vi "Instrument Sequence.vi"(0 "Function":T5=enum."Initialize Dialog", 1 "Caller VI":enum16{"User", "Stress Measurement VI"}(ring), 2 "Which Program?":T1, 5 "Notifiers":T8, 7 "Message Queues":T21, 9 "Refnums":T6, 11 "error in (no error)":errorcluster, 12 "Configuration":variant) -> (8 "Instrument Steps":T2, 15 "error out":errorcluster)   [LabVIEW 2014]
uses:
  support/Message Queue/All Message Queues.ctl
  support/Message Queue/Message Cluster.ctl
  support/Notifiers/Notifiers.ctl
  support/Message Handler Loop Notifiers.ctl
  Hardware Control/Parameter Analyzer/Parameter Analyzer Notifiers.ctl
  Hardware Control/Switching Matrix/Switching Matrix Notifiers.ctl
  Hardware Control/Stress Control/StressControl Notifiers.ctl
  Hardware Control/Spectrometer/Spectrometer Notifiers.ctl
  Hardware Control/Switches and Mirrors/SwitchesMirrors Notifiers.ctl
  Hardware Control/Camera/Camera Notifiers.ctl
  Hardware Control/XYZ Stage/XYZ Notifications.ctl
  Hardware Control/Autofocus/Autofocus Notifiers.ctl
  Optoelectronic Measurement/Optoelectronic Notifiers.ctl
  Save Data/SaveData Notifiers.ctl
  Instrument Sequence Notifiers.ctl
  Instrument Sequence Refnums.ctl
  Action.ctl
  Instrument List.ctl
  Plot Data/Electrical Data Plot Refnums.ctl
  Instrument Sequence Function.ctl
  Instrument Steps.ctl
  Instrument Stequence - Which Program.ctl
  support/Status of All Instruments.ctl
  Hardware Control/Parameter Analyzer/Parameter Analyzer Data.ctl
  Hardware Control/Parameter Analyzer/Parameter Analyzer Config.ctl
  Hardware Control/Parameter Analyzer/Parameter Analyzer Integration Parameters.ctl
  Hardware Control/Parameter Analyzer/Parameter Analyzer SMU Sweeping.ctl
  Hardware Control/Parameter Analyzer/Parameter Analyzer Sweep Spacing.ctl
  Hardware Control/Parameter Analyzer/Parameter Analyzer SMU Range.ctl
  Hardware Control/Parameter Analyzer/Parameter Analyzer SMU Sampling.ctl
  Hardware Control/Parameter Analyzer/Parameter Analyzer Sampling Parameters.ctl
  Hardware Control/Parameter Analyzer/Parameter Analyzer Stop Sampling Conditions.ctl
  Hardware Control/Parameter Analyzer/Parameter Analyzer Refnums.ctl
  Hardware Control/Parameter Analyzer/Parameter Analyzer Initialization.ctl
  Hardware Control/Switching Matrix/Switching Matrix Data.ctl
  Hardware Control/Switching Matrix/Switching Matrix Config.ctl
  Hardware Control/Switching Matrix/Switching Matrix Refnums.ctl
  Hardware Control/Switching Matrix/Switching Matrix Initialization.ctl
  Hardware Control/Stress Control/StressControl Data.ctl
  Hardware Control/Stress Control/StressControl Config.ctl
  Hardware Control/Stress Control/StressControl Refnums.ctl
  Hardware Control/Stress Control/StressControl Initialization.ctl
  Hardware Control/Spectrometer/Spectrometer Data.ctl
  Hardware Control/Spectrometer/Spectrometer Config.ctl
  Hardware Control/Spectrometer/Laser Settings.ctl
  Hardware Control/Spectrometer/Laser.ctl
  Hardware Control/Spectrometer/Filter.ctl
  Hardware Control/Spectrometer/Grating Detector Settings.ctl
  Hardware Control/Spectrometer/Grating.ctl
  Hardware Control/Spectrometer/Detector.ctl
  Hardware Control/Spectrometer/Acquisition Settings.ctl
  Hardware Control/Spectrometer/Spectrometer Refnum.ctl
  Plot Data/Optical Spectrum Plot Refnum.ctl
  Hardware Control/Spectrometer/Spectrometer Initialization.ctl
  Hardware Control/Switches and Mirrors/SwitchesMirrors Data.ctl
  Hardware Control/Switches and Mirrors/SwitchesMirrors Config.ctl
  Hardware Control/Switches and Mirrors/SwitchesMirrors Status.ctl
  Hardware Control/Switches and Mirrors/SwitchesMirrors Refnum.ctl
  Hardware Control/Switches and Mirrors/SwitchesMirrors Initialize.ctl
  Hardware Control/Camera/Camera Data.ctl
  Hardware Control/Camera/Camera Config.ctl
  Hardware Control/Camera/Camera Settings.ctl
  Hardware Control/Camera/Camera Refnums.ctl
  Hardware Control/Camera/Camera Initialization.ctl
  Hardware Control/XYZ Stage/XYZ Data.ctl
  Hardware Control/XYZ Stage/XYZ Config.ctl
  Hardware Control/XYZ Stage/XYZ Connection Settings.ctl
  Hardware Control/XYZ Stage/XYZ Stage Control.ctl
  Hardware Control/XYZ Stage/XYZ Coordinate Control.ctl
  Hardware Control/XYZ Stage/XYZ Refnums.ctl
  Hardware Control/XYZ Stage/XYZ Initialization.ctl
  Hardware Control/Autofocus/AutoFocus Data.ctl
  Hardware Control/Autofocus/AutoFocus Config.ctl
  Hardware Control/Autofocus/ZScan.ctl
  <vilib>/Analysis/Matrix/Datatypes/RealMatrix.ctl
  Hardware Control/Autofocus/AutoFocus Refnums.ctl
  Hardware Control/Autofocus/Target Refnums.ctl
  Hardware Control/Autofocus/AutoFocus Initialize.ctl
  Hardware Control/Parameter Analyzer/Electrical Data.ctl
  Plot Data/WhichInstrument.ctl
  Hardware Control/Spectrometer/Spectral Data.ctl
  Optoelectronic Measurement/Optoelectronic Measurement.ctl
  <vilib>/Utility/sysdir.llb/System Directory Type.ctl
  support/Message Queue/Message Queue.lvlib
  <vilib>/Analysis/Matrix/NI_Matrix.lvlib
panel:
  out "Device Info":string
  out "Device Name":string
  # "LICENSED MATERIALS – PROPERTY OF IBM\nCopyright IBM Corp. 2016,\nALL RIGHTS RESERVED"
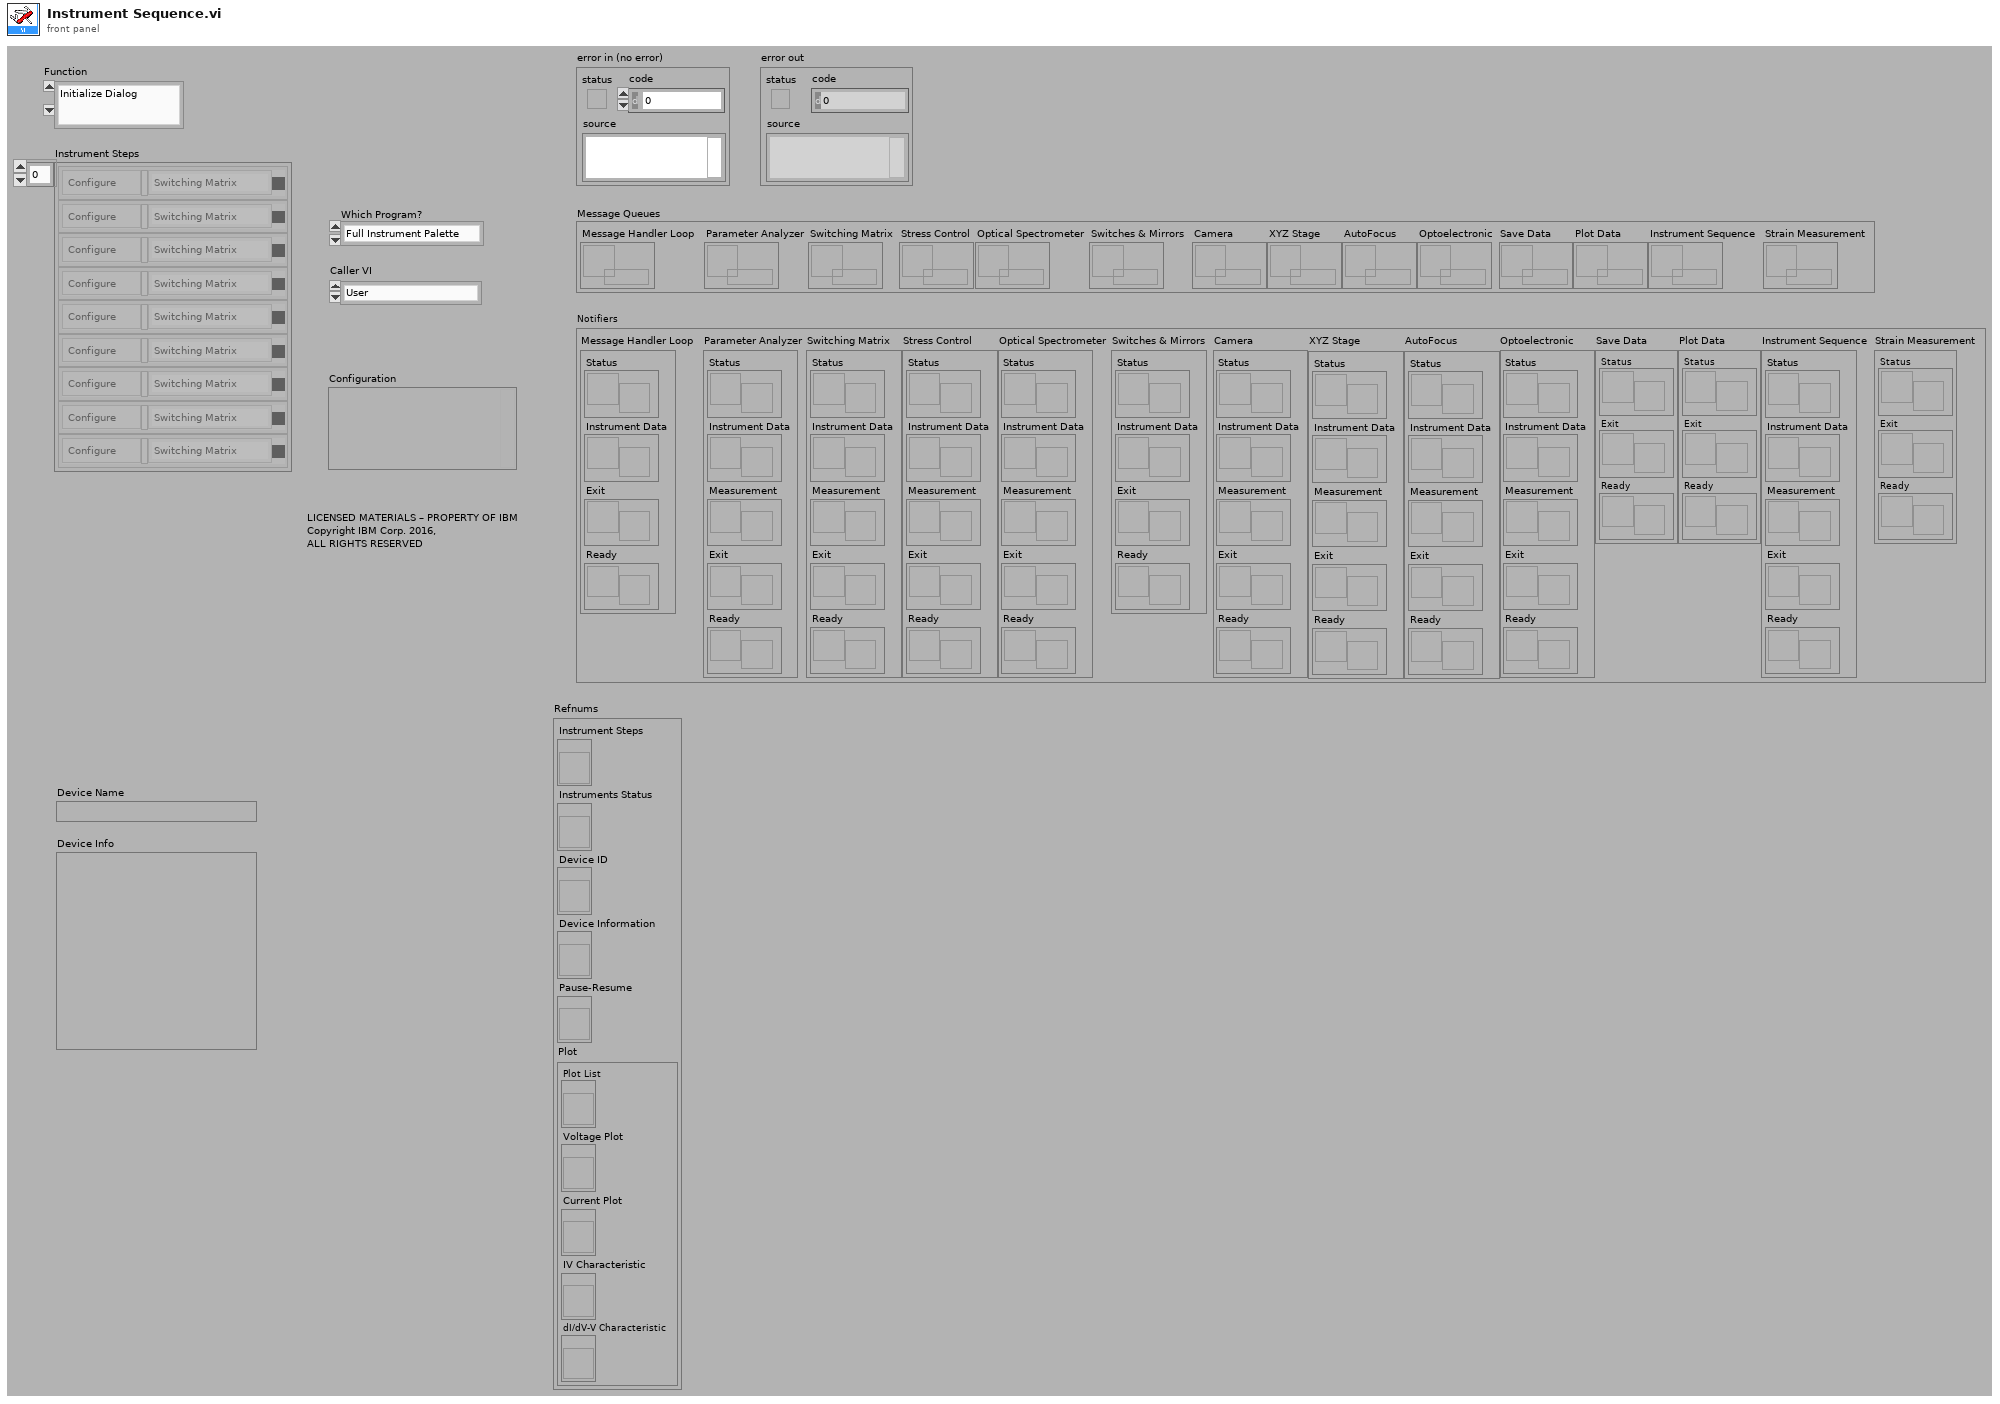
[diagram p1: front panel]
types:
  T1 = typedef "Instrument Stequence - Which Program.ctl" = enum16{"Full Instrument Palette", "Strain Electrical"}
  T2 = typedef "Instrument Steps.ctl" = cluster{"Action":T3, "Configuration":variant, "Instrument":T4, "Status":enum8{"False", "True", "Mixed"}}[]
  T3 = typedef "Action.ctl" = enum32{"Configure", "Measure"}
  T4 = typedef "Instrument List.ctl" = enum32{"Unknown Instrument", "Switching Matrix", "Parameter Analyzer", "Optical Spectrometer", "Optoelectronic", "Autofocus"}
  T5 = typedef "Instrument Sequence Function.ctl" = enum16{"Update Refnums", "Get Instruments Status", "Initialize Dialog", "Get Autofocus Status", "Add Step", "Remove Step", "Clear Sequence", "Load Sequence", "Save Sequence", "Measure Sequence", "Reset Sequence", "Start Sequence", "Start Sequence for Strain Measurement", "Stop Sequence", "Pause Sequence", "Update Sequence Status", "Choose What Next", "Update Workspace Data", "Save Measured Sequence", "Configure Parameter Analyzer", "Perform Electrical Measurement", "Configure Switching Matrix", "Configure Optical Spectrometer", "Focus", "Perform Optical Measurement", "Perform Optoelectronic Measurement", "Declare Completion"}
  T6 = typedef "Instrument Sequence Refnums.ctl" = cluster{"Instrument Steps":refnum<vi>, "Instruments Status":refnum<vi>, "Device ID":refnum<vi>, "Device Information":refnum<vi>, "Pause-Resume":refnum<vi>, "Plot":T7}
  T7 = typedef "Electrical Data Plot Refnums.ctl" = cluster{"Plot List":refnum<vi>, "Voltage Plot":refnum<vi>, "Current Plot":refnum<vi>, "IV Characteristic":refnum<vi>, "dI/dV-V Characteristic":refnum<vi>}
  T8 = typedef "Notifiers.ctl" = cluster{"Message Handler Loop":T9, "Parameter Analyzer":T10, "Switching Matrix":T11, "Stress Control":T12, "Optical Spectrometer":T13, "Switches & Mirrors":T14, "Camera":T15, "XYZ Stage":T16, "AutoFocus":T17, "Optoelectronic":T18, "Save Data":T19, "Plot Data":T19, "Instrument Sequence":T20, "Strain Measurement":cluster{"Status":refnum<notifier>, "Exit":refnum<notifier>, "Ready":refnum<notifier>}}
  T9 = typedef "Message Handler Loop Notifiers.ctl" = cluster{"Status":refnum<notifier>, "Instrument Data":refnum<notifier>, "Exit":refnum<notifier>, "Ready":refnum<notifier>}
  T10 = typedef "Parameter Analyzer Notifiers.ctl" = cluster{"Status":refnum<notifier>, "Instrument Data":refnum<notifier>, "Measurement":refnum<notifier>, "Exit":refnum<notifier>, "Ready":refnum<notifier>}
  T11 = typedef "Switching Matrix Notifiers.ctl" = cluster{"Status":refnum<notifier>, "Instrument Data":refnum<notifier>, "Measurement":refnum<notifier>, "Exit":refnum<notifier>, "Ready":refnum<notifier>}
  T12 = typedef "StressControl Notifiers.ctl" = cluster{"Status":refnum<notifier>, "Instrument Data":refnum<notifier>, "Measurement":refnum<notifier>, "Exit":refnum<notifier>, "Ready":refnum<notifier>}
  T13 = typedef "Spectrometer Notifiers.ctl" = cluster{"Status":refnum<notifier>, "Instrument Data":refnum<notifier>, "Measurement":refnum<notifier>, "Exit":refnum<notifier>, "Ready":refnum<notifier>}
  T14 = typedef "SwitchesMirrors Notifiers.ctl" = cluster{"Status":refnum<notifier>, "Instrument Data":refnum<notifier>, "Exit":refnum<notifier>, "Ready":refnum<notifier>}
  T15 = typedef "Camera Notifiers.ctl" = cluster{"Status":refnum<notifier>, "Instrument Data":refnum<notifier>, "Measurement":refnum<notifier>, "Exit":refnum<notifier>, "Ready":refnum<notifier>}
  T16 = typedef "XYZ Notifications.ctl" = cluster{"Status":refnum<notifier>, "Instrument Data":refnum<notifier>, "Measurement":refnum<notifier>, "Exit":refnum<notifier>, "Ready":refnum<notifier>}
  T17 = typedef "Autofocus Notifiers.ctl" = cluster{"Status":refnum<notifier>, "Instrument Data":refnum<notifier>, "Measurement":refnum<notifier>, "Exit":refnum<notifier>, "Ready":refnum<notifier>}
  T18 = typedef "Optoelectronic Notifiers.ctl" = cluster{"Status":refnum<notifier>, "Instrument Data":refnum<notifier>, "Measurement":refnum<notifier>, "Exit":refnum<notifier>, "Ready":refnum<notifier>}
  T19 = typedef "SaveData Notifiers.ctl" = cluster{"Status":refnum<notifier>, "Exit":refnum<notifier>, "Ready":refnum<notifier>}
  T20 = typedef "Instrument Sequence Notifiers.ctl" = cluster{"Status":refnum<notifier>, "Instrument Data":refnum<notifier>, "Measurement":refnum<notifier>, "Exit":refnum<notifier>, "Ready":refnum<notifier>}
  T21 = typedef "Message Queue.lvlib/All Message Queues.ctl" = cluster{"Message Handler Loop":refnum<queue>, "Parameter Analyzer":refnum<queue>, "Switching Matrix":refnum<queue>, "Stress Control":refnum<queue>, "Optical Spectrometer":refnum<queue>, "Switches & Mirrors":refnum<queue>, "Camera":refnum<queue>, "XYZ Stage":refnum<queue>, "AutoFocus":refnum<queue>, "Optoelectronic":refnum<queue>, "Save Data":refnum<queue>, "Plot Data":refnum<queue>, "Instrument Sequence":refnum<queue>, "Strain Measurement":refnum<queue>}
  T22 = typedef "WhichInstrument.ctl" = enum16{"No Plot", "Spectrometer", "Parameter Analyzer", "Optoelectronic"}
  T23 = typedef "Electrical Data.ctl" = cluster{"Sequence":dbl[], "V1":dbl[], "V2":dbl[], "V3":dbl[], "V4":dbl[], "I1":dbl[], "I2":dbl[], "I3":dbl[], "I4":dbl[]}
  T24 = typedef "Spectral Data.ctl" = cluster{"Intensity":dbl[], "Wavelength":dbl[], "Energy":dbl[], "Raman Shift":dbl[], "Detector Temperature":dbl}
  T25 = typedef "Optoelectronic Measurement.ctl" = cluster{"Optical Spectrum":T24, "Electrical Measurement":T23}
  T26 = typedef "Parameter Analyzer Data.ctl" = cluster{"Configuration":T27, "Refnums":T35, "Initialization":T36}
  T27 = typedef "Parameter Analyzer Config.ctl" = cluster{"Parameter Analyzer VISA Session":refnum<visa-resource-name>, "Sweeping Time Parameters":T28, "Acquisition Mode":enum32{"Sweeping Mode", "Sampling Mode"}, "Status Polling Time (ms)":u32, "Comment":string, "SMU 1 - Sweeping":T29, "SMU 2 - Sweeping":T29, "SMU 3 - Sweeping":T29, "SMU 4 - Sweeping":T29, "Sweep Spacing":T30, "Range":T31, "SMU1 - Sampling":T32, "SMU2 - Sampling":T32, "SMU3 - Sampling":T32, "SMU4 - Sampling":T32, "Sampling Time Parameters":T33, "Stop Condition":T34}
  T28 = typedef "Parameter Analyzer Integration Parameters.ctl" = cluster{"Integration Time":u32, "Short Integration Time (s)":dbl, "Long Integration Time (s)":dbl, "Wait Time Parameter":dbl}
  T29 = typedef "Parameter Analyzer SMU Sweeping.ctl" = cluster{"Start / Offset":dbl, "Stop / Ratio":dbl, "Step \n(linear only)":dbl, "Compliance":dbl, "Power \nCompliance":dbl, "Mode":u32, "Function":i32, "Sweep Mode":bool}
  T30 = typedef "Parameter Analyzer Sweep Spacing.ctl" = u16
  T31 = typedef "Parameter Analyzer SMU Range.ctl" = u16
  T32 = typedef "Parameter Analyzer SMU Sampling.ctl" = cluster{"Source":dbl, "Compliance":dbl, "Mode":u32, "Function":bool}
  T33 = typedef "Parameter Analyzer Sampling Parameters.ctl" = cluster{"Initial Interval (s)":dbl, "Number of Samples":i32, "Total Sampling Time (s)":dbl, "Hold Time (s)":dbl, "Sampling Mode":i32, "Sampling Time":i32}
  T34 = typedef "Parameter Analyzer Stop Sampling Conditions.ctl" = cluster{"Enable Delay (s)":dbl, "Name":string, "Threshold":dbl, "num. of events":i32, "Event":i32, "Stop Condition Enable":bool}
  T35 = typedef "Parameter Analyzer Refnums.ctl" = cluster{"Status":refnum<vi>, "Electrical Measurement":refnum<vi>, "Plots":T7, "HP Integration Time":refnum<vi>, "VISA":refnum<vi>, "Sweeping Time Parameters":refnum<vi>, "Acquisition Mode":refnum<vi>, "SMU 1 - Sweeping":refnum<vi>, "SMU 2 - Sweeping":refnum<vi>, "SMU 3 - Sweeping":refnum<vi>, "SMU 4 - Sweeping":refnum<vi>, "Sweep Spacing":refnum<vi>, "Range":refnum<vi>, "SMU1 - Sampling":refnum<vi>, "SMU2 - Sampling":refnum<vi>, "SMU3 - Sampling":refnum<vi>, "SMU4 - Sampling":refnum<vi>, "Sampling Time Parameters":refnum<vi>, "Stop Condition":refnum<vi>, "Instrument Status":refnum<vi>}
  T36 = typedef "Parameter Analyzer Initialization.ctl" = cluster{"Update Visa Session":bool, "Configure Integration Time":bool, "Configure Acquisition Mode":bool, "Update Refnums":bool}
  T37 = typedef "Switching Matrix Data.ctl" = cluster{"Configuration":T38, "Refnums":T39, "Initialization":T40}
  T38 = typedef "Switching Matrix Config.ctl" = cluster{"Switching Matrix VISA Session":refnum<visa-resource-name>, "Connections":cluster{"Connections":bool[], "Connection Type":enum16{"Disconnected", "Make - Break", "Break - Make"}}[]}
  T39 = typedef "Switching Matrix Refnums.ctl" = cluster{"Connections":refnum<vi>, "Instrument Status":refnum<vi>}
  T40 = typedef "Switching Matrix Initialization.ctl" = cluster{"Update Visa Session":bool, "Update Refnums":bool}
  T41 = typedef "Spectrometer Data.ctl" = cluster{"Configuration":T42, "Refnums":T50, "Initialization":T52}
  T42 = typedef "Spectrometer Config.ctl" = cluster{"Laser Settings":T43, "Spectrometer Settings":T46, "Acquisition Settings":T49, "Path":path}
  T43 = typedef "Laser Settings.ctl" = cluster{"Laser Wavelength":T44, "Neutral Density Filter":T45}
  T44 = typedef "Laser.ctl" = enum16{"633 nm", "784 nm", "532 nm", "365 nm"}
  T45 = typedef "Filter.ctl" = enum16{"100%", "50%", "25%", "10%", "1%", "0.1%", "0.01%"}
  T46 = typedef "Grating Detector Settings.ctl" = cluster{"Confocal Hole Size (µm)":dbl, "Grating":T47, "Detector":T48}
  T47 = typedef "Grating.ctl" = u16
  T48 = typedef "Detector.ctl" = enum16{"InGaAs Array", "Silicon CCD"}
  T49 = typedef "Acquisition Settings.ctl" = cluster{"Acquisition Mode":enum16{"Single Window", "Multi-Window"}, "Spectal Position (nm)":dbl, "From (nm)":dbl, "To (nm)":dbl, "Integration Time (s)":dbl, "Number of Accumulations":i32, "AutoScanning":bool, "Spike Removal":bool}
  T50 = typedef "Spectrometer Refnum.ctl" = cluster{"Instrument Status":refnum<vi>, "Optical Spectrum Plot":T51, "Laser":refnum<vi>, "Filter":refnum<vi>, "Laser ON?":refnum<vi>, "Hole":refnum<vi>, "Grating":refnum<vi>, "Detector":refnum<vi>, "Acquisition Mode":refnum<vi>, "Spectal Position":refnum<vi>, "From":refnum<vi>, "To":refnum<vi>, "Integration Time":refnum<vi>, "Accumulations":refnum<vi>, "AutoScanning":refnum<vi>, "Spike Removal":refnum<vi>, "Acquisition Mode Panel":refnum<vi>}
  T51 = typedef "Optical Spectrum Plot Refnum.ctl" = cluster{"Plot List":refnum<vi>, "Optical Spectrum vs Energy":refnum<vi>, "Optical Spectrum vs Wavelength":refnum<vi>, "Optical Spectrum vs Raman Shift":refnum<vi>, "Detector Temperature":refnum<vi>}
  T52 = typedef "Spectrometer Initialization.ctl" = cluster{"Connect":bool, "Update Refnums":bool, "Get Configuration":bool}
  T53 = typedef "AutoFocus Data.ctl" = cluster{"Configuration":T54, "Refnums":T57, "Initialize":T59}
  T54 = typedef "AutoFocus Config.ctl" = cluster{"Matching Criteria":cluster{"Minimum Score":sgl, "Color Score Weight":sgl, "Minimum Contrast":i32, "Match Mode":u32, "Match Feature Mode":u32, "Subpixel Accuracy":bool, "Color Sensitivity":u32, "Search Strategy":u32}, "Z Scan Parameters":T55, "Displacement":dbl, "Transformation Matrix":T56}
  T55 = typedef "ZScan.ctl" = cluster{"Z Range":ext, "Resolution":dbl, "Initial Direction":enum16{"Up", "Down"}, "Focus Threshold":dbl, "Ascent Constant":dbl}
  T56 = typedef "NI_Matrix.lvlib/RealMatrix.ctl" = dbl[][]
  T57 = typedef "AutoFocus Refnums.ctl" = cluster{"Instrument Status":refnum<vi>, "Matching Criteria":refnum<vi>, "Z Scan Parameters":refnum<vi>, "Distance":refnum<vi>, "Transformation Matrix":refnum<vi>, "Match and Edge":T58, "Matching Curves":refnum<vi>, "Tracking":refnum<vi>, "Focus":refnum<vi>, "Find Focus":refnum<vi>, "Set Target":refnum<vi>, "Link Stage & Camera":refnum<vi>, "Align":refnum<vi>}
  T58 = typedef "Target Refnums.ctl" = cluster{"Image":refnum<vi>, "Target":refnum<vi>, "Edge":refnum<vi>, "Target Data":refnum<vi>}
  T59 = typedef "AutoFocus Initialize.ctl" = cluster{"Update Refnums":bool, "Allocate Image Memory":bool, "Set Match Criteria":bool, "Link Stage & Camera":bool, "Set Target":bool, "Find Target":bool}
  T60 = typedef "Status of All Instruments.ctl" = cluster{"Parameter Analyzer":T26, "Swithing Matrix":T37, "Stress Control":T61, "Optical Spectrometer":T41, "Switches & Mirrors":T65, "Camera":T70, "XYZ Stage":T75, "AutoFocus":T53}
  T61 = typedef "StressControl Data.ctl" = cluster{"Configuration":T62, "Refnums":T63, "Initialization":T64}
  T62 = typedef "StressControl Config.ctl" = cluster{"Stress Control VISA Session":refnum<visa-resource-name>, "Axis":i32, "Motion":u16, "Destination (°)":dbl, "Speed (°/s)":dbl, "Position (°)":dbl}
  T63 = typedef "StressControl Refnums.ctl" = cluster{"Instrument Status":refnum<vi>, "Position":refnum<vi>, "Mecahnism Motion":refnum<vi>, "Destination":refnum<vi>, "Apply Stress":refnum<vi>, "Stop":refnum<vi>, "Stress Control VISA":refnum<vi>}
  T64 = typedef "StressControl Initialization.ctl" = cluster{"Update Visa Session":bool, "Update Configuration":bool, "Update Refnums":bool, "Get Position":bool}
  T65 = typedef "SwitchesMirrors Data.ctl" = cluster{"Configuration":T66, "Refnums":T68, "Initialize":T69}
  T66 = typedef "SwitchesMirrors Config.ctl" = cluster{"Relay VISA Session":refnum<visa-resource-name>, "Switches":T67, "Delays (ms)":cluster{"Laser":u32, "Video":u32}}
  T67 = typedef "SwitchesMirrors Status.ctl" = cluster{"Laser":bool, "Video":bool}
  T68 = typedef "SwitchesMirrors Refnum.ctl" = cluster{"Instrument Status":refnum<vi>, "Laser":refnum<vi>, "Video":refnum<vi>, "Relay VISA":refnum<vi>}
  T69 = typedef "SwitchesMirrors Initialize.ctl" = cluster{"Update Refnums":bool, "Connect":bool, "Set Configuration":bool}
  T70 = typedef "Camera Data.ctl" = cluster{"Configuration":T71, "Refnums":T73, "Initialization":T74}
  T71 = typedef "Camera Config.ctl" = cluster{"Settings":T72}
  T72 = typedef "Camera Settings.ctl" = cluster{"Pixel clock":i32, "Frame rate":dbl, "Exposure time":dbl, "Master Gain":i32, "Red Gain":i32, "Green Gain":i32, "Blue Gain":i32, "Auto Gain":bool, "White-balance":bool, "Color Correction":bool}
  T73 = typedef "Camera Refnums.ctl" = cluster{"Pixel Clock":refnum<vi>, "Frame Rate":refnum<vi>, "Exposure Time":refnum<vi>, "Master Gain":refnum<vi>, "Red Gain":refnum<vi>, "Green Gain":refnum<vi>, "Blue Gain":refnum<vi>, "Auto Gain":refnum<vi>, "Auto White-balance":refnum<vi>, "Color Correction":refnum<vi>, "Image":refnum<vi>, "Video Button":refnum<vi>, "Instrument Status":refnum<vi>}
  T74 = typedef "Camera Initialization.ctl" = cluster{"Connect":bool, "Update Refnums":bool, "Acquiring?":bool}
  T75 = typedef "XYZ Data.ctl" = cluster{"Configuration":T76, "Refnums":T80, "Initialization":T81}
  T76 = typedef "XYZ Config.ctl" = cluster{"Connection Settings":T77, "Manual Control":T78, "Coordinate Control":T79}
  T77 = typedef "XYZ Connection Settings.ctl" = cluster{"Tango VISA":refnum<visa-resource-name>, "Baudrate":i32, "Show Protocol?":bool}
  T78 = typedef "XYZ Stage Control.ctl" = cluster{"North":bool, "South":bool, "West":bool, "East":bool, "Up":bool, "Down":bool, "Stop":bool, "XY Step":dbl, "Z step":dbl}
  T79 = typedef "XYZ Coordinate Control.ctl" = cluster{"Motion Mode":enum16{"Absolute", "Relative"}, "Destination [mm]":dbl[]}
  T80 = typedef "XYZ Refnums.ctl" = cluster{"Instrument Status":refnum<vi>, "Position":refnum<vi>, "Manual Control":refnum<vi>, "Up":refnum<vi>, "Down":refnum<vi>, "North":refnum<vi>, "South":refnum<vi>, "East":refnum<vi>, "West":refnum<vi>, "Stop":refnum<vi>, "Limits":refnum<vi>}
  T81 = typedef "XYZ Initialization.ctl" = cluster{"Update Visa Session":bool, "Set To Default":bool, "Get Status":bool, "Update Refnums":bool}
  T82 = typedef "System Directory Type.ctl" = i32
  T83 = cluster{"Action":T3, "Configuration":variant, "Instrument":T4, "Status":enum8{"False", "True", "Mixed"}}
  T84 = typedef "SaveData Workspace Info.ctl" = cluster{"Device Name":string, "Device Info":string, "Path":path}
  T85 = typedef "Measurement.ctl" = cluster{"Which Instrument?":T22, "Electrical Measurement":T23, "Measurement Mode":enum16{"Sweeping Mode", "Sampling Mode"}, "Optical Spectrum":T24}
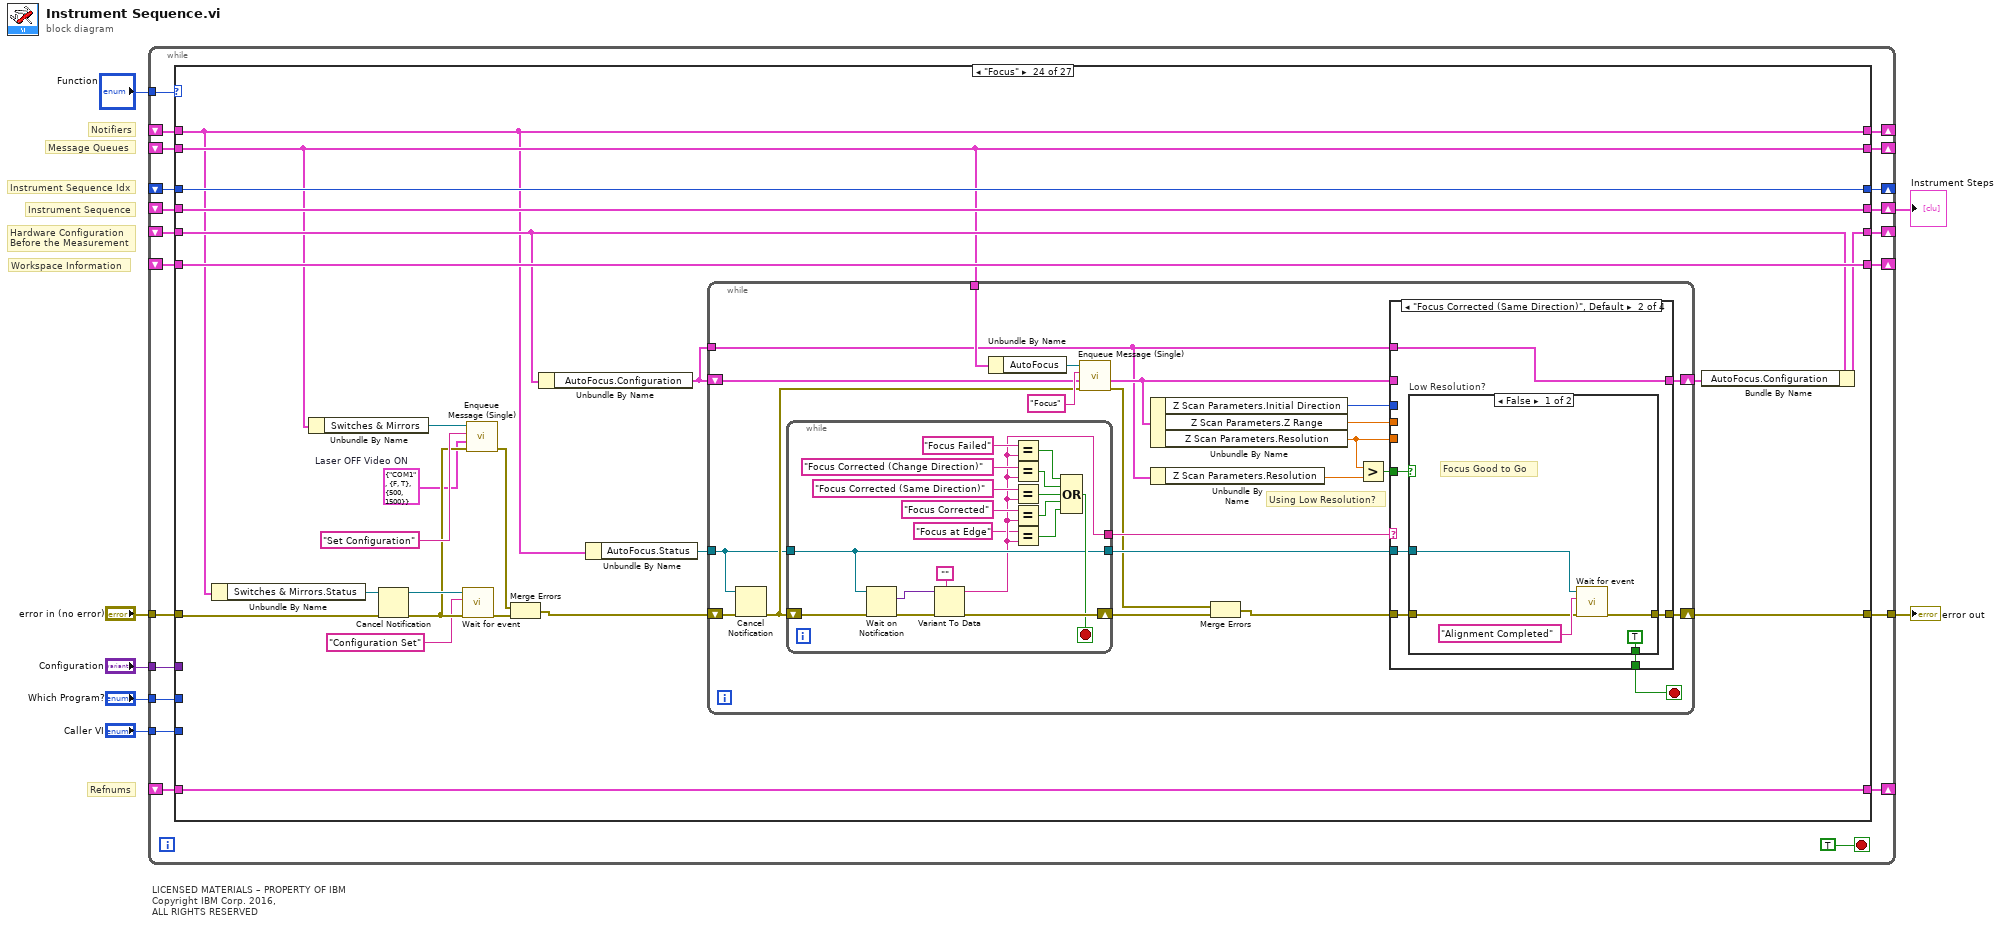
[diagram p0: block diagram]
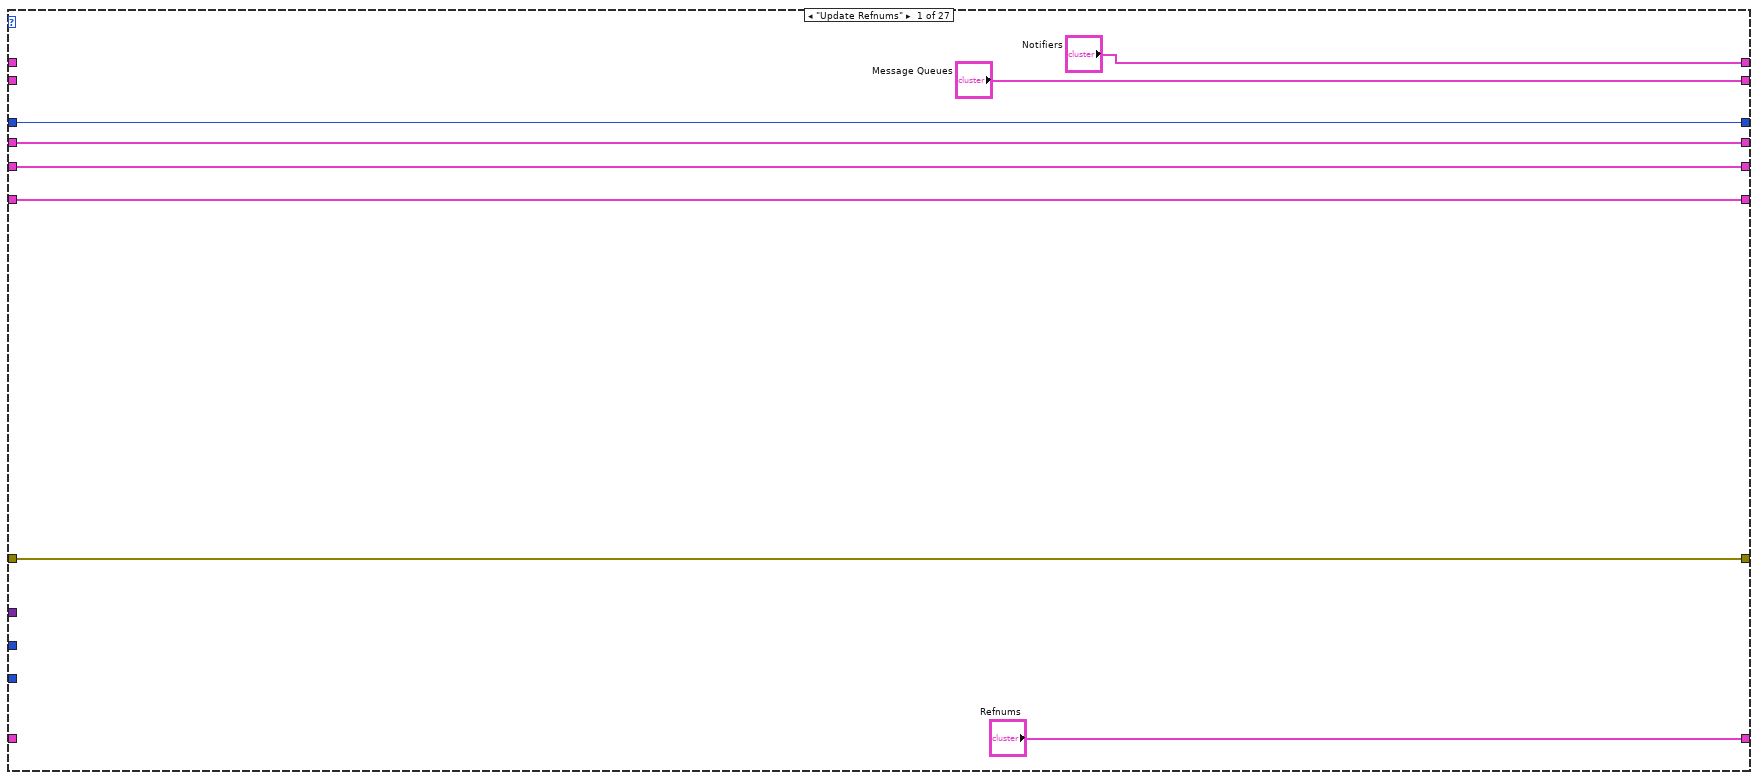
[diagram p2: hidden frame]
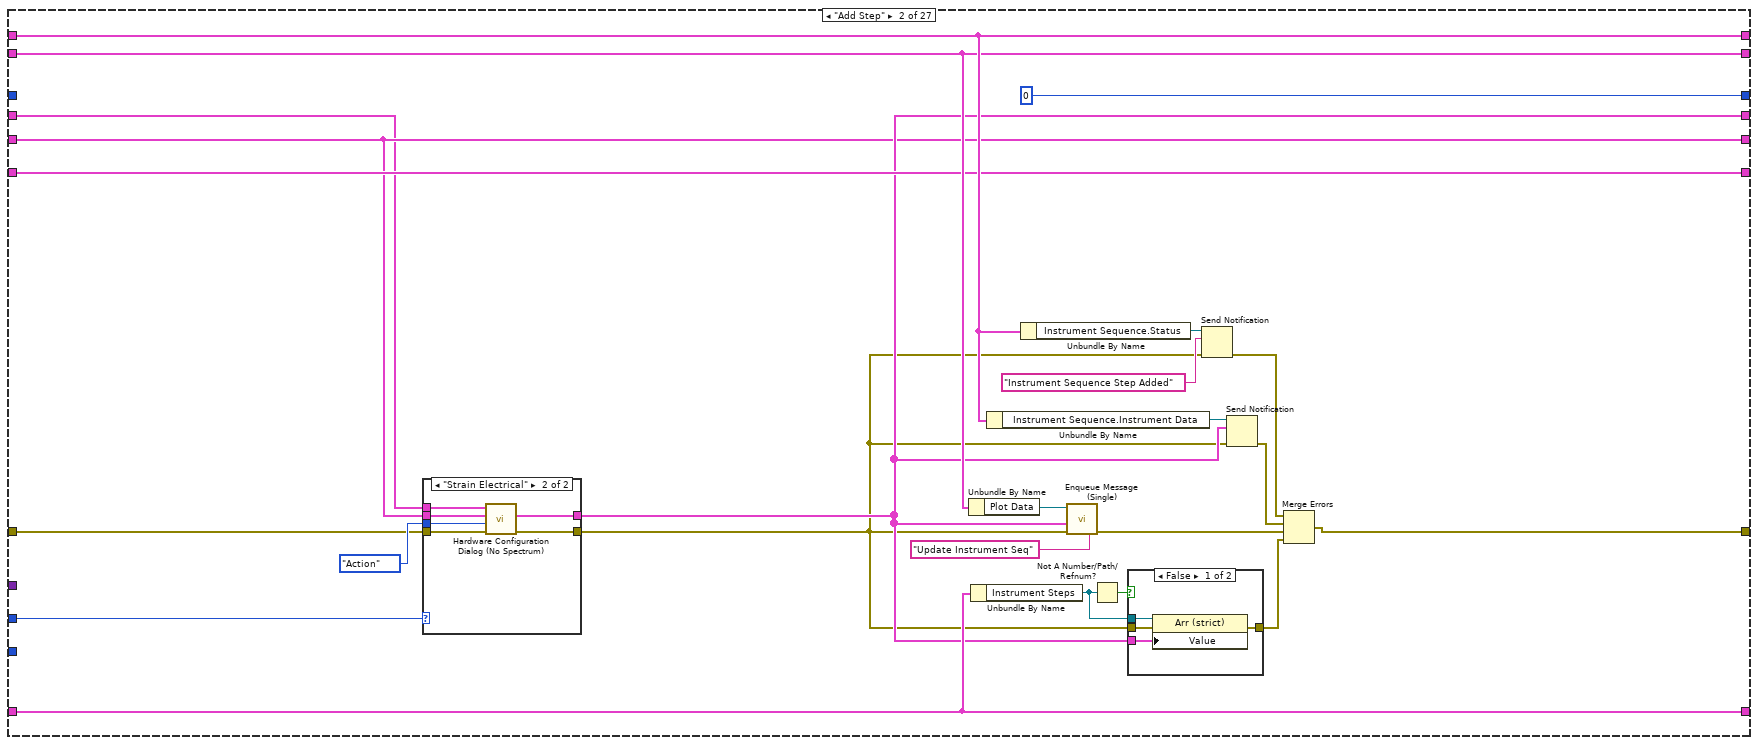
[diagram p3: hidden frame]
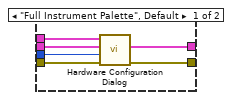
[diagram p4: hidden frame]
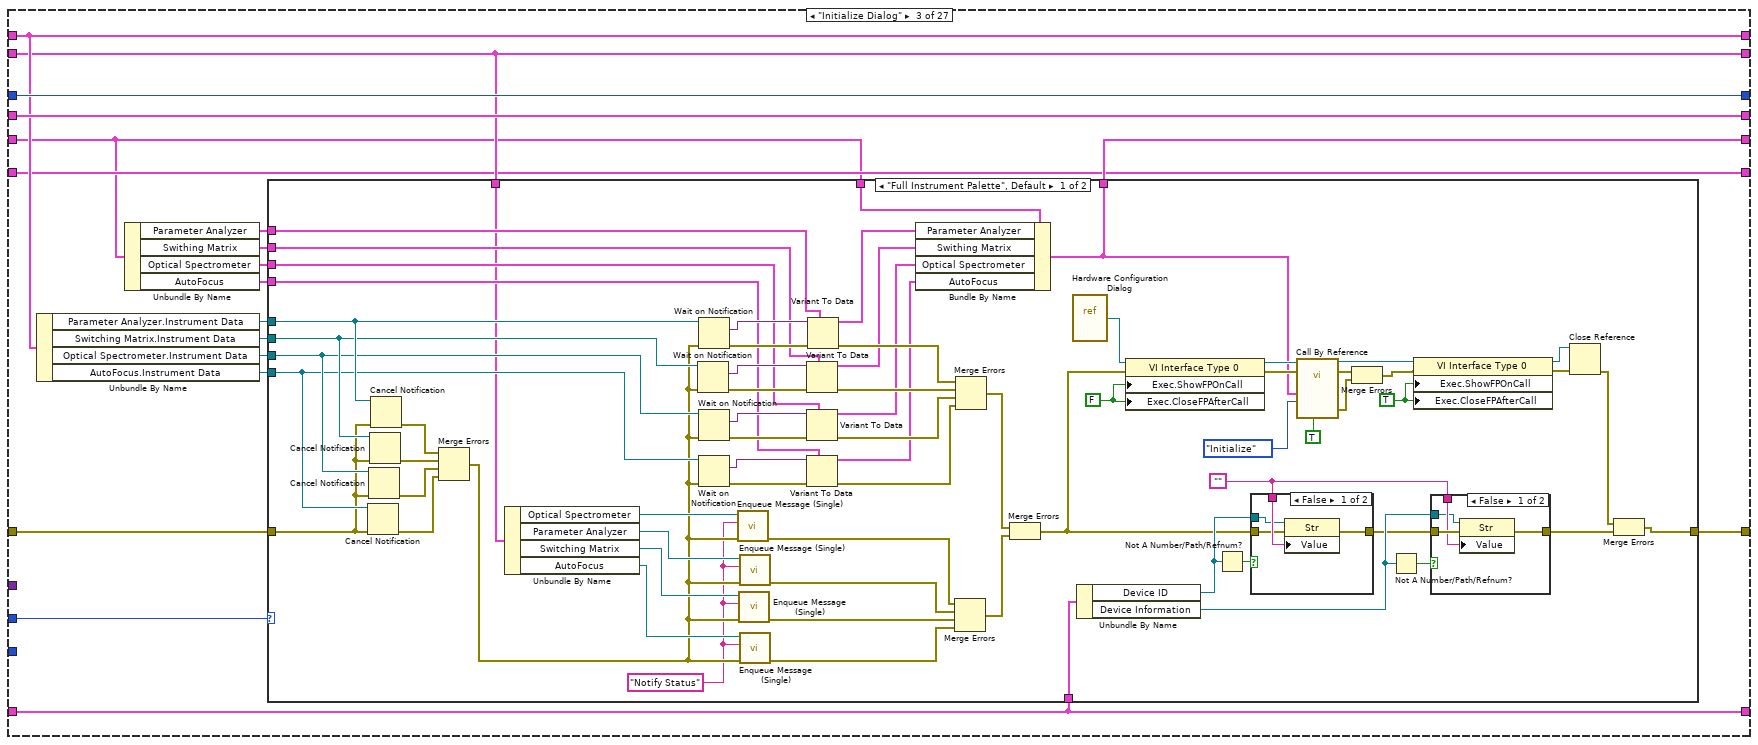
[diagram p6: hidden frame]
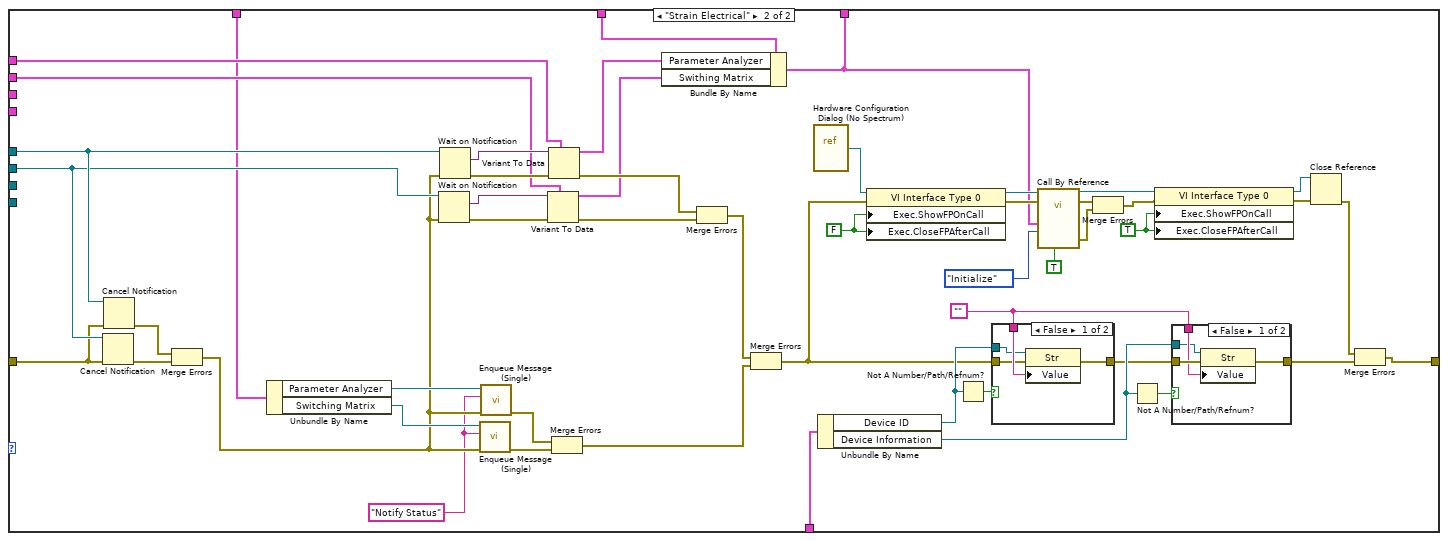
[diagram p9: hidden frame]
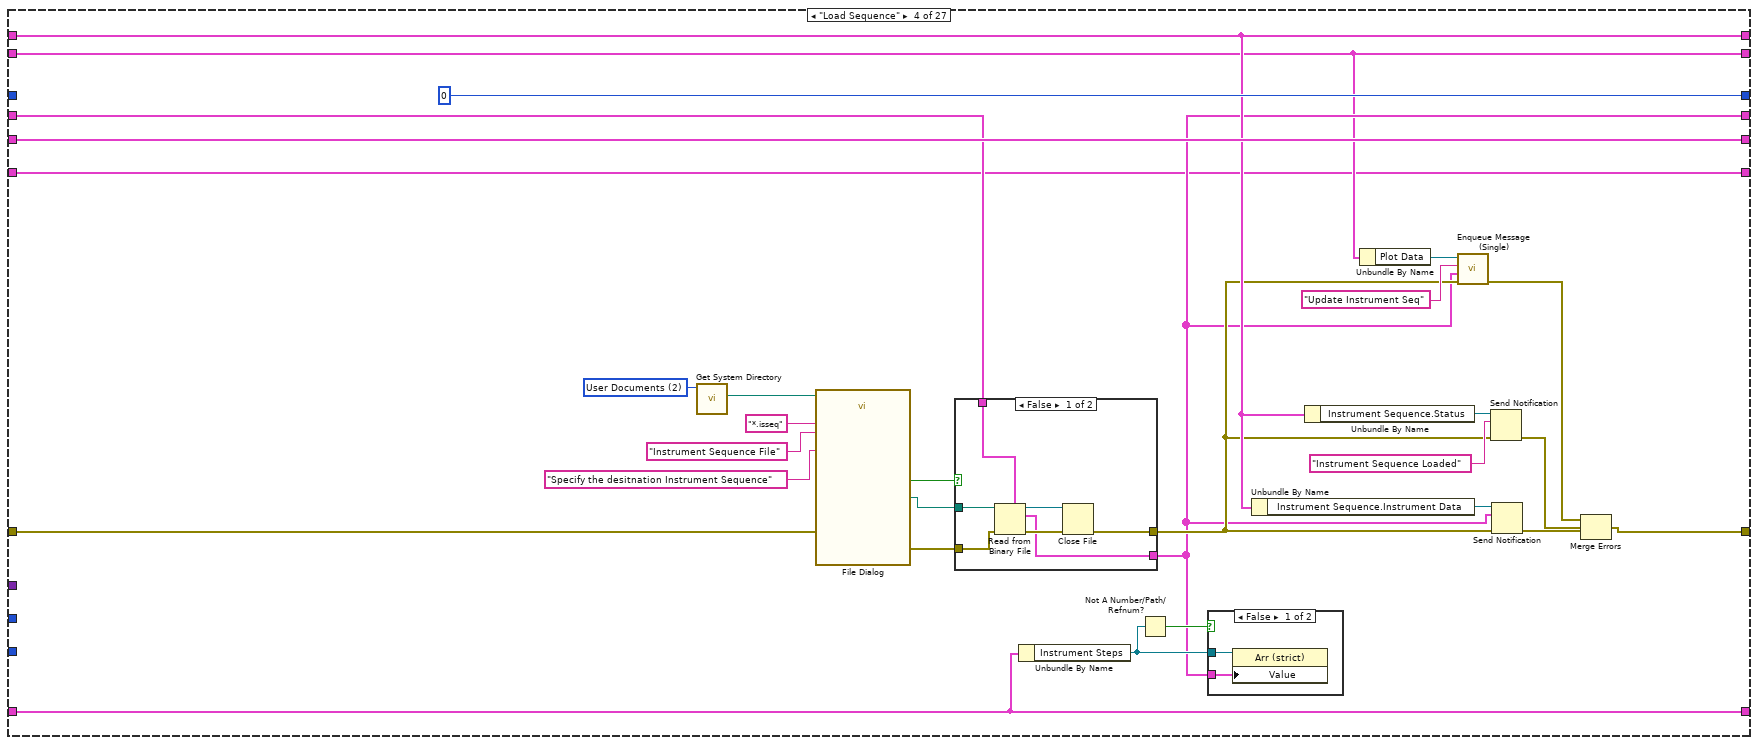
[diagram p12: hidden frame]
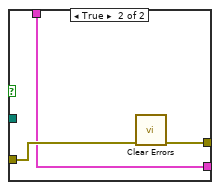
[diagram p13: hidden frame]
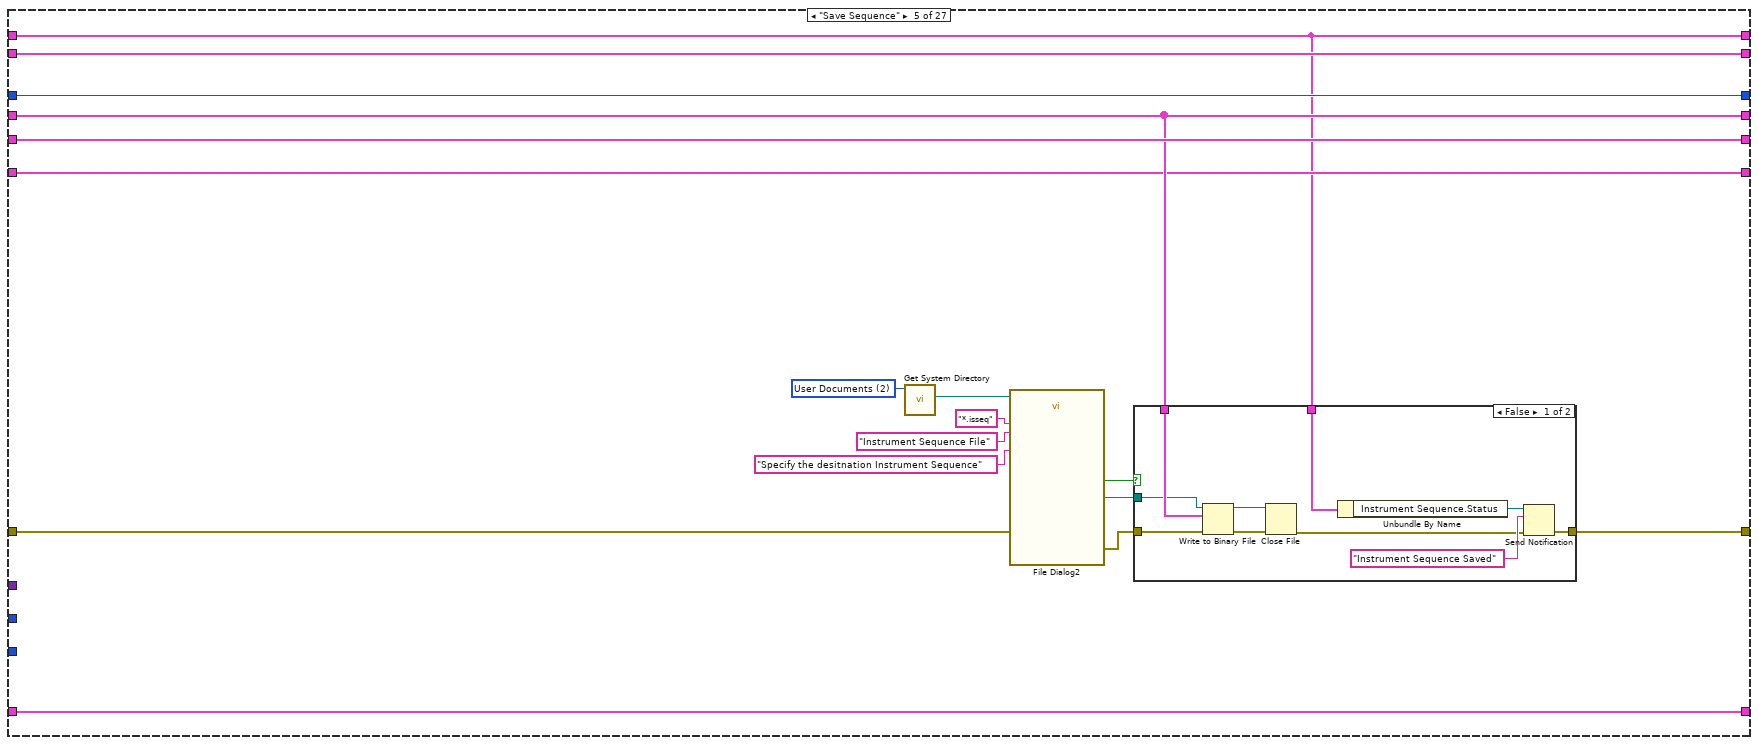
[diagram p15: hidden frame]
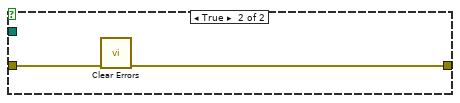
[diagram p16: hidden frame]
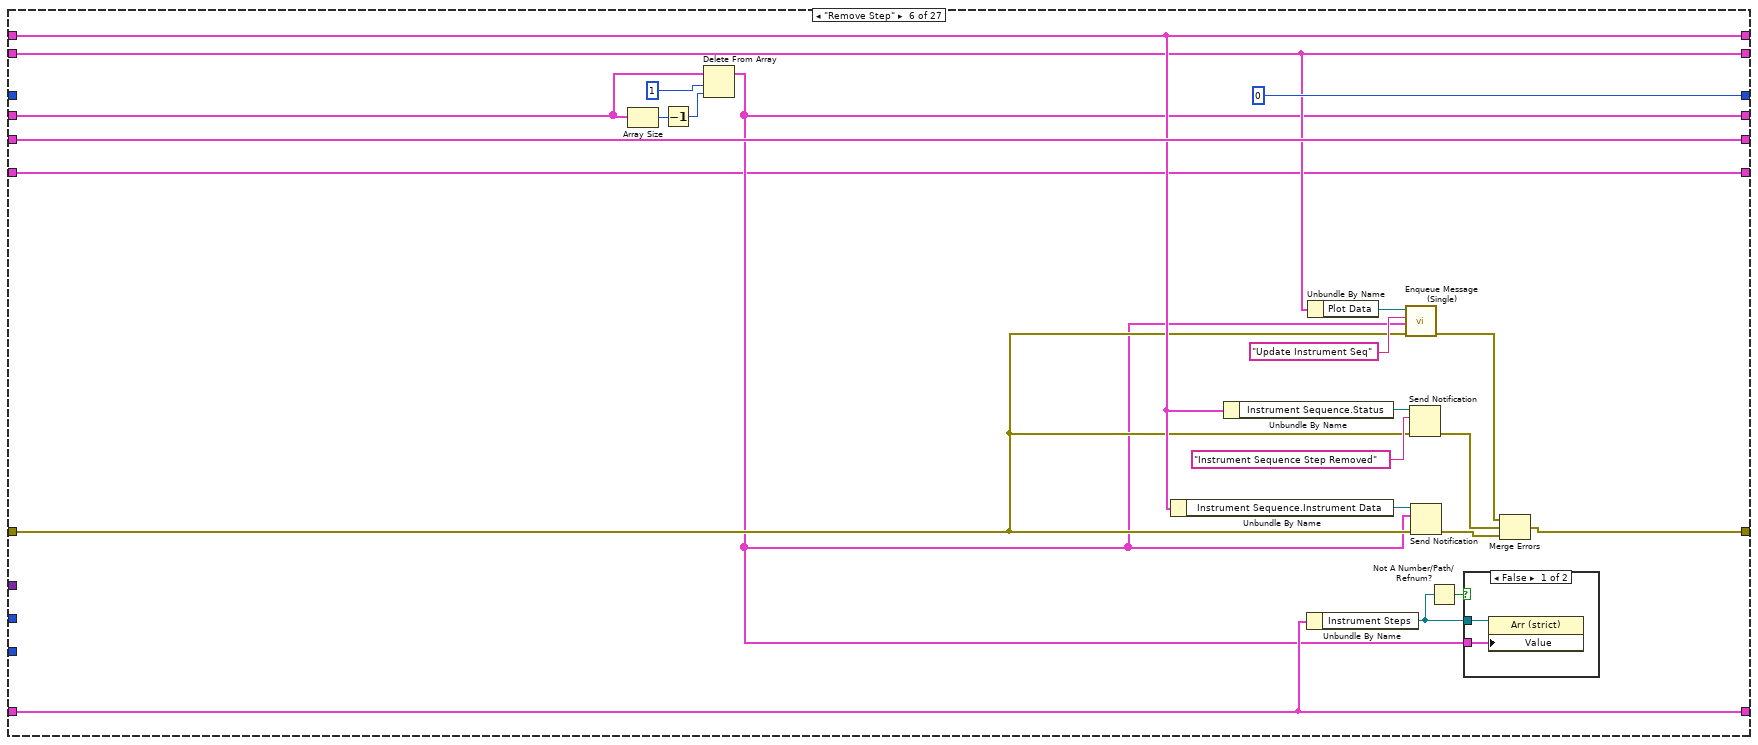
[diagram p17: hidden frame]
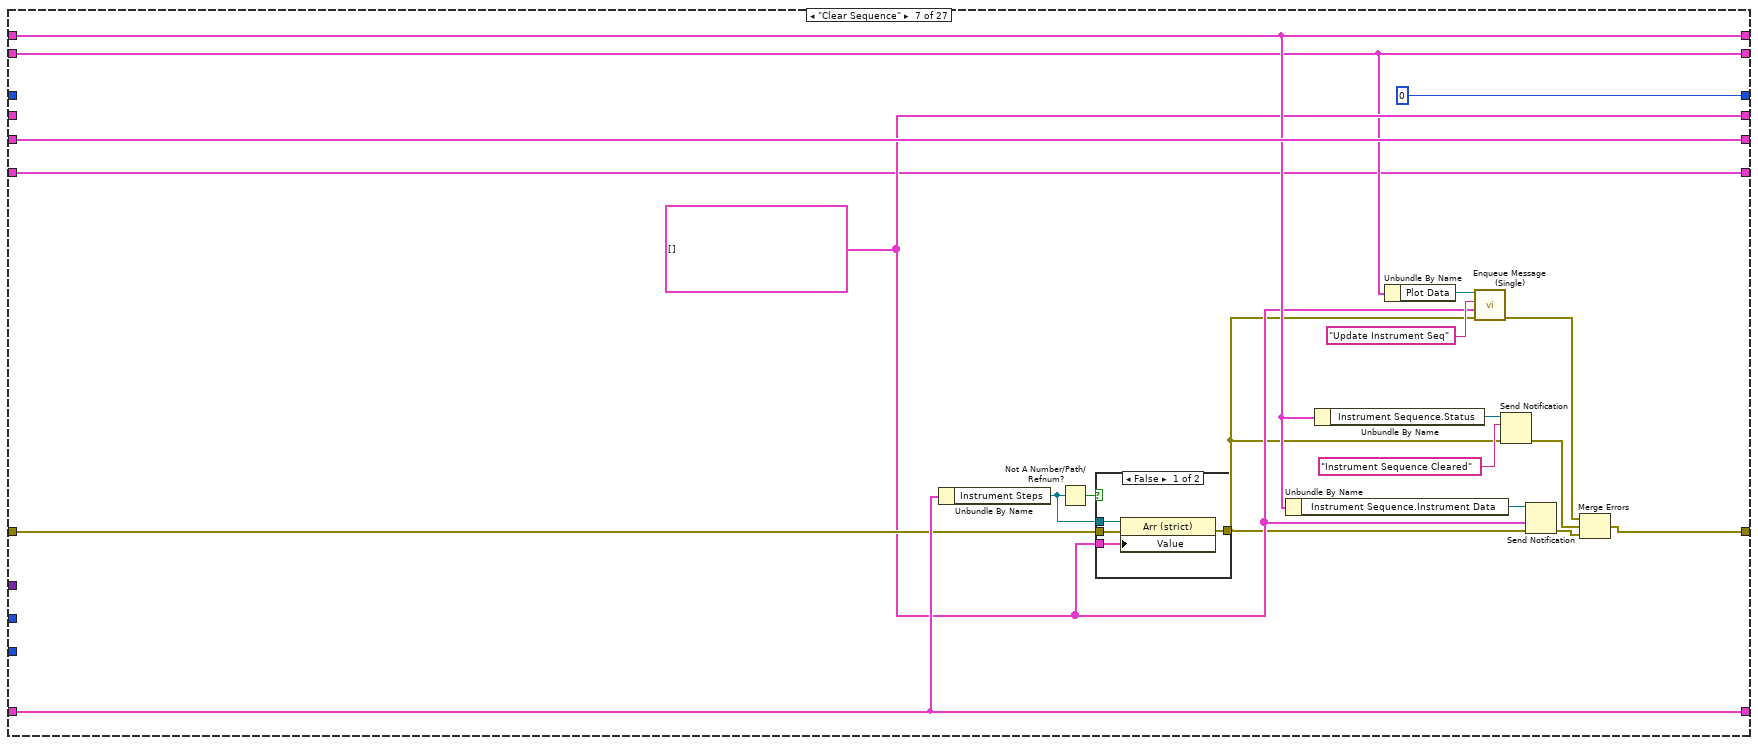
[diagram p19: hidden frame]
diagram:
  # "LICENSED MATERIALS – PROPERTY OF IBM\nCopyright IBM Corp. 2016,\nALL RIGHTS RESERVED"
  # "Workspace Information"
  # "Instrument Sequence Idx"
  # "Instrument Sequence"
  # "Refnums"
  # "Hardware Configuration\nBefore the Measurement"
  # "Message Queues"
  # "Notifiers"
  n1 = while {
    tunnel: "error in (no error)" -> [w28]
    tunnel: [w27] -> w6
    tunnel: "Function" -> [w26]
    shift-right: [w21] -> _
    shift-left: _ -> [w22]
    shift-right: [w20] -> _
    shift-left: _ -> [w25]
    shift-right: [w19] -> _
    shift-left: _ -> [w24]
    shift-right: [w17] -> _
    shift-left: _ -> [w18]
    shift-right: [w16] -> w4
    shift-left: _ -> [w15]
    shift-right: [w13] -> _
    shift-left: _ -> [w14]
    tunnel: "Configuration" -> [w12]
    tunnel: "Caller VI" -> [w11]
    shift-right: [w9] -> _
    shift-left: _ -> [w10]
    tunnel: "Which Program?" -> [w8]
    stop <- TRUE stop-if-true
    n2 = case shown="\"Focus\"" w26 {
      tunnel: w28 -> [w36 w38 w82 w256 w284 w307 w339 w380 w388 w408 w481 w519 w550 w597 w631 w648 w749 w763 w816 w897 w957 w993 w1024 w1057 w1170 w1179 w1189]
      tunnel: [w36 w44 w93 w246 w278 w314 w340 w372 w387 w411 w487 w513 w551 w593 w627 w661 w738 w776 w835 w914 w967 w1005 w1041 w1049 w1165 w1177 w1190] -> w27
      tunnel: w25 -> [_ w51 w83 w249 w279 w315 w341 w359 w400 w421 w486 w512 w540 w598 w633 w659 w754 w790 w832 w911 w969 w987 w1018 w1050 w1174 w1184 w1187]
      tunnel: w24 -> [_ w48 w81 w238 w291 w309 w334 w358 w391 w406 w496 w526 w544 w590 w642 w658 w753 w765 w834 w913 w965 w1003 w1039 w1051 w1168 w1183 w1197]
      tunnel: ["Refnums" w57 w94 w260 w290 w323 w345 w386 w401 w422 w483 w522 w546 w594 w638 w660 w755 w796 w865 w940 w968 w1007 w1043 w1068 w1169 w1178 w1193] -> w21
      tunnel: w22 -> [_ w57 w94 w260 w290 w323 w345 w386 w401 w422 w483 w522 w546 w594 w638 w660 w755 w796 w865 w940 w968 w1007 w1043 w1068 w1169 w1178 w1193]
      tunnel: ["Notifiers" w51 w83 w249 w279 w315 w341 w359 w400 w421 w486 w512 w540 w598 w633 w659 w754 w790 w832 w911 w969 w987 w1018 w1050 w1174 w1184 w1187] -> w20
      tunnel: ["Message Queues" w48 w81 w238 w291 w309 w334 w358 w391 w406 w496 w526 w544 w590 w642 w658 w753 w765 w834 w913 w965 w1003 w1039 w1051 w1168 w1183 w1197] -> w19
      tunnel: w18 -> [w32 w40 w79 w263 w292 w327 w349 w385 w399 w420 w494 w525 w541 w587 w641 _ w741 w778 w805 w889 w974 w1011 w1046 w1054 w1171 w1180 w1194]
      tunnel: [w32 w40 w84 w263 w292 w327 w349 w385 w399 w420 w494 w525 w541 w587 w641 w657 w752 w778 w805 w889 w961 w1000 w1036 w1053 w1171 w1180 w1194] -> w17
      tunnel: [w30 w43 w96 w242 w288 w306 w336 w384 w398 w419 w482 w511 w545 w589 w639 w652 w751 w795 w863 w938 w977 w1012 w1047 w1070 w1172 w1181 w1195] -> w16
      tunnel: w15 -> [w30 w39 w96 w253 w288 w319 _ w384 w398 w419 w495 w510 w545 w589 w639 w652 w751 w795 w863 w938 w977 w1012 w1047 w1070 w1172 w1181 w1195]
      tunnel: w14 -> [w31 _ w95 _ w289 _ _ w383 w397 w418 _ w509 w548 _ w640 w651 w750 w794 w862 w937 w978 w1013 w1048 w1071 w1173 w1182 w1196]
      tunnel: [w31 0 w95 0 w289 0 0 w383 w397 w418 0 w509 w547 0 w640 w651 w750 w794 w862 w937 w978 w1013 w1048 w1071 w1173 w1182 w1196] -> w13
      tunnel: w12 -> [_ _ _ _ _ _ _ _ _ _ _ _ _ _ _ _ _ _ _ _ w966 w1006 w1042 _ _ _ _]
      tunnel: w11 -> [_ _ _ _ _ _ _ _ _ w402 _ _ w543 _ _ _ _ _ _ _ _ _ _ _ _ _ w1188]
      tunnel: w10 -> [w29 w47 w80 w237 w280 w305 w330 w379 w395 w403 w479 w505 w542 _ w635 w644 w742 w775 w833 w912 w959 w999 w1029 w1067 w1166 w1175 w1185]
      tunnel: [w29 w47 w80 w237 w280 w305 w330 w379 w395 w403 w479 w505 w542 w588 w635 w644 w742 w775 w833 w912 w959 w999 w1029 w1067 w1166 w1175 w1185] -> w9
      tunnel: w8 -> [_ w37 w78 _ _ _ _ _ _ _ _ _ _ _ _ w643 _ _ _ _ _ _ _ _ _ _ _]
      frame "Update Refnums" {
      }
      frame "Add Step" {
        n3 = case shown="\"Strain Electrical\"" w37 {
          tunnel: [w66 w72] -> w43
          tunnel: [w65 w71] -> w42
          tunnel: enum16{"Initialize", "Action"}."Action" ("Function") -> [w64 w70]
          tunnel: w40 -> [w63 w69]
          tunnel: w39 -> [w62 w68]
          tunnel: w38 -> [w61 w67]
          frame "Full Instrument Palette", Default {
            n4 = call "Hardware Configuration Dialog.vi"("error in (no error)"=w61, "Function"=w64, "Hardware Status"=w63, "Instrument Steps In"=w62) -> ("error out"=w65:errorcluster, "Instrument Steps Out"=w66:T2)  [unwired: 6 in]
          }
          frame "Strain Electrical" {
            n5 = call "Hardware Configuration Dialog (No Spectrum).vi"("error in (no error)"=w67, "Function"=w70, "Hardware Status"=w69, "Instrument Steps In"=w68) -> ("error out"=w71:errorcluster, "Instrument Steps Out"=w72:T2)  [unwired: 6 in]
          }
        }
        n6 = Unbundle By Name(w48) -> ("Plot Data"=w50:refnum<queue>)
        n7 = Unbundle By Name(w57) -> ("Instrument Steps"=w58:refnum<vi>)
        n8 = Unbundle By Name(w51) -> ("Instrument Sequence.Instrument Data"=w54:refnum<notifier>)
        n9 = Unbundle By Name(w51) -> ("Instrument Sequence.Status"=w55:refnum<notifier>)
        n10 = call "Enqueue Message (Single).vi"("error in (no error)"=w42, "Message Data"=w43, "Message"="Update Instrument Seq", "Message Queue"=w50) -> ("error out"=w45:errorcluster)  [unwired: 7 out]
        n11 = Not A Number/Path/Refnum?(number/path/refnum=w58) -> (NaN/Path/Refnum?=w59:bool)
        n12 = case shown="False" w59 {
          tunnel: w58 -> [w76 _]
          tunnel: w43 -> [w75 _]
          tunnel: w42 -> [w74 w77]
          tunnel: [w73 w77] -> w46
          frame False {
            n13 = property class="Arr (strict)"(reference=w76, error in=w74, "Value"=w75) -> (error out=w73:errorcluster)  [unwired: 1 out]
          }
          frame True {
          }
        }
        n14 = Send Notification(notification="Instrument Sequence Step Added", notifier=w55, error in (no error)=w42) -> (error out=w52:errorcluster)  [unwired: 1 out]
        n15 = Send Notification(notification=w43, notifier=w54, error in (no error)=w42) -> (error out=w53:errorcluster)  [unwired: 1 out]
        n16 = Merge Errors(w52, w53, w45, w46) -> (w44:errorcluster)
      }
      frame "Initialize Dialog" {
        n17 = Unbundle By Name(w83) -> ("Parameter Analyzer.Instrument Data"=w90:refnum<notifier>, "Switching Matrix.Instrument Data"=w89:refnum<notifier>, "Optical Spectrometer.Instrument Data"=w88:refnum<notifier>, "AutoFocus.Instrument Data"=w86:refnum<notifier>)
        n18 = Unbundle By Name(w79) -> ("Parameter Analyzer"=w92:T26, "Swithing Matrix"=w91:T37, "Optical Spectrometer"=w87:T41, "AutoFocus"=w85:T53)
        n19 = case shown="\"Full Instrument Palette\", Default" w78 {
          tunnel: w94 -> [w158 w218]
          tunnel: [w143 w203] -> w93
          tunnel: w92 -> [w134 w195]
          tunnel: w91 -> [w133 w194]
          tunnel: w90 -> [w131 w192]
          tunnel: w89 -> [w130 w191]
          tunnel: w88 -> [w119 _]
          tunnel: w87 -> [w118 _]
          tunnel: w86 -> [w114 _]
          tunnel: w85 -> [w111 _]
          tunnel: [w97 w175] -> w84
          tunnel: w82 -> [w101 w179]
          tunnel: w81 -> [w100 w178]
          tunnel: w79 -> [w98 w176]
          frame "Full Instrument Palette", Default {
            w104 = "Notify Status" ("Message")
            w149 = TRUE ("Execution:Show Front Panel On Call")
            w150 = FALSE ("Execution:Show Front Panel On Call")
            w157 = "" ("Device Name")
            n20 = Cancel Notification(0:w114, 3:w101) -> (11:w115:errorcluster)  [unwired: 2 out]
            n21 = Cancel Notification(0:w119, 3:w101) -> (11:w123:errorcluster)  [unwired: 2 out]
            n22 = Cancel Notification(0:w130, 3:w101) -> (11:w129:errorcluster)  [unwired: 2 out]
            n23 = Cancel Notification(0:w131, 3:w101) -> (11:w128:errorcluster)  [unwired: 2 out]
            n24 = Merge Errors(w128, w129, w123, w115) -> (w105:errorcluster)
            n25 = Unbundle By Name(w100) -> ("Optical Spectrometer"=w109:refnum<queue>, "Parameter Analyzer"=w108:refnum<queue>, "Switching Matrix"=w107:refnum<queue>, "AutoFocus"=w106:refnum<queue>)
            n26 = Wait on Notification(notifier=w130, error in (no error)=w105) -> (notification=w135:variant, error out=w136:errorcluster)  [unwired: 4 out]
            n27 = Wait on Notification(notifier=w131, error in (no error)=w105) -> (notification=w141:variant, error out=w140:errorcluster)  [unwired: 4 out]
            n28 = Wait on Notification(notifier=w119, error in (no error)=w105) -> (notification=w120:variant, error out=w122:errorcluster)  [unwired: 4 out]
            n29 = Wait on Notification(notifier=w114, error in (no error)=w105) -> (notification=w113:variant, error out=w112:errorcluster)  [unwired: 4 out]
            n30 = call "Enqueue Message (Single).vi"("error in (no error)"=w105, "Message"=w104, "Message Queue"=w109) -> ("error out"=w103:errorcluster)  [unwired: 1 in, 7 out]
            n31 = call "Enqueue Message (Single).vi"("error in (no error)"=w105, "Message"=w104, "Message Queue"=w107) -> ("error out"=w138:errorcluster)  [unwired: 1 in, 7 out]
            n32 = call "Enqueue Message (Single).vi"("error in (no error)"=w105, "Message"=w104, "Message Queue"=w108) -> ("error out"=w139:errorcluster)  [unwired: 1 in, 7 out]
            n33 = call "Enqueue Message (Single).vi"("error in (no error)"=w105, "Message"=w104, "Message Queue"=w106) -> ("error out"=w137:errorcluster)  [unwired: 1 in, 7 out]
            n34 = Variant To Data(error in=w136, type=w133, Variant=w135) -> (data=w116:T37, error out=w126:errorcluster)
            n35 = Variant To Data(error in=w122, type=w118, Variant=w120) -> (data=w117:T41, error out=w121:errorcluster)
            n36 = Variant To Data(error in=w112, type=w111, Variant=w113) -> (data=w102:T53, error out=w110:errorcluster)
            n37 = Variant To Data(error in=w140, type=w134, Variant=w141) -> (data=w132:T26, error out=w127:errorcluster)
            n38 = Bundle By Name(cluster=w98, "Parameter Analyzer"=w132, "Swithing Matrix"=w116, "Optical Spectrometer"=w117, "AutoFocus"=w102) -> (w97:T60)
            n39 = Merge Errors(w103, w139, w138, w137) -> (w124:errorcluster)
            n40 = Merge Errors(w127, w126, w121, w110) -> (w125:errorcluster)
            n41 = Merge Errors(w125, w124) -> (w99:errorcluster)
            n42 = vi-ref "Hardware Configuration Dialog.vi"() -> (w148:refnum<vi>)
            n43 = Unbundle By Name(w158) -> ("Device ID"=w162:refnum<vi>, "Device Information"=w164:refnum<vi>)
            n44 = property class="VI Interface Type 0"(reference=w148, error in=w99, "Exec.ShowFPOnCall"=w150, "Exec.CloseFPAfterCall"=w150) -> (reference out=w144:refnum<vi>, error out=w145:errorcluster)
            n45 = Not A Number/Path/Refnum?(number/path/refnum=w162) -> (NaN/Path/Refnum?=w161:bool)
            n46 = case shown="False" w161 {
              tunnel: [w173 w174] -> w160
              tunnel: w157 -> [w172 _]
              tunnel: w162 -> [w171 _]
              tunnel: w99 -> [w170 w174]
              frame False {
                n47 = property class="Str"(reference=w171, error in=w170, "Value"=w172) -> (error out=w173:errorcluster)  [unwired: 1 out]
              }
              frame True {
              }
            }
            n48 = call-by-ref "?"(reference=w144, error in=w145, "Update UI Values?"=TRUE, "Function"=enum16{"Initialize", "Action"}."Initialize", "Hardware Status"=w97) -> (reference out=w147:refnum<vi>, error out=w153:errorcluster, 0:"error out"=w156:errorcluster)  [unwired: 7 in, 1 out]
            n49 = Merge Errors(w153, w156) -> (w146:errorcluster)
            n50 = Not A Number/Path/Refnum?(number/path/refnum=w164) -> (NaN/Path/Refnum?=w163:bool)
            n51 = property class="VI Interface Type 0"(reference=w147, error in=w146, "Exec.ShowFPOnCall"=w149, "Exec.CloseFPAfterCall"=w149) -> (reference out=w151:refnum<vi>, error out=w152:errorcluster)
            n52 = case shown="False" w163 {
              tunnel: w160 -> [w168 w169]
              tunnel: [w167 w169] -> w159
              tunnel: w157 -> [w166 _]
              tunnel: w164 -> [w165 _]
              frame False {
                n53 = property class="Str"(reference=w165, error in=w168, "Value"=w166) -> (error out=w167:errorcluster)  [unwired: 1 out]
              }
              frame True {
              }
            }
            n54 = Close Reference(reference=w151, error in (no error)=w152) -> (error out=w142:errorcluster)
            n55 = Merge Errors(w142, w159) -> (w143:errorcluster)
          }
          frame "Strain Electrical" {
            w180 = "Notify Status" ("Message")
            w209 = TRUE ("Execution:Show Front Panel On Call")
            w210 = FALSE ("Execution:Show Front Panel On Call")
            w217 = "" ("Device Name")
            n56 = Cancel Notification(0:w191, 3:w179) -> (11:w190:errorcluster)  [unwired: 2 out]
            n57 = Cancel Notification(0:w192, 3:w179) -> (11:w189:errorcluster)  [unwired: 2 out]
            n58 = Merge Errors(w189, w190) -> (w181:errorcluster)
            n59 = Unbundle By Name(w178) -> ("Parameter Analyzer"=w183:refnum<queue>, "Switching Matrix"=w182:refnum<queue>)
            n60 = Wait on Notification(notifier=w191, error in (no error)=w181) -> (notification=w196:variant, error out=w197:errorcluster)  [unwired: 4 out]
            n61 = Wait on Notification(notifier=w192, error in (no error)=w181) -> (notification=w201:variant, error out=w200:errorcluster)  [unwired: 4 out]
            n62 = call "Enqueue Message (Single).vi"("error in (no error)"=w181, "Message"=w180, "Message Queue"=w182) -> ("error out"=w198:errorcluster)  [unwired: 1 in, 7 out]
            n63 = call "Enqueue Message (Single).vi"("error in (no error)"=w181, "Message"=w180, "Message Queue"=w183) -> ("error out"=w199:errorcluster)  [unwired: 1 in, 7 out]
            n64 = Variant To Data(error in=w197, type=w194, Variant=w196) -> (data=w184:T37, error out=w187:errorcluster)
            n65 = Variant To Data(error in=w200, type=w195, Variant=w201) -> (data=w193:T26, error out=w188:errorcluster)
            n66 = Merge Errors(w199, w198) -> (w185:errorcluster)
            n67 = Bundle By Name(cluster=w176, "Parameter Analyzer"=w193, "Swithing Matrix"=w184) -> (w175:T60)
            n68 = Merge Errors(w188, w187) -> (w186:errorcluster)
            n69 = Merge Errors(w186, w185) -> (w177:errorcluster)
            n70 = vi-ref "Hardware Configuration Dialog (No Spectrum).vi"() -> (w208:refnum<vi>)
            n71 = Unbundle By Name(w218) -> ("Device ID"=w222:refnum<vi>, "Device Information"=w224:refnum<vi>)
            n72 = property class="VI Interface Type 0"(reference=w208, error in=w177, "Exec.ShowFPOnCall"=w210, "Exec.CloseFPAfterCall"=w210) -> (reference out=w204:refnum<vi>, error out=w205:errorcluster)
            n73 = Not A Number/Path/Refnum?(number/path/refnum=w222) -> (NaN/Path/Refnum?=w221:bool)
            n74 = case shown="False" w221 {
              tunnel: [w233 w234] -> w220
              tunnel: w217 -> [w232 _]
              tunnel: w222 -> [w231 _]
              tunnel: w177 -> [w230 w234]
              frame False {
                n75 = property class="Str"(reference=w231, error in=w230, "Value"=w232) -> (error out=w233:errorcluster)  [unwired: 1 out]
              }
              frame True {
              }
            }
            n76 = call-by-ref "?"(reference=w204, error in=w205, "Update UI Values?"=TRUE, "Function"=enum16{"Initialize", "Action"}."Initialize", "Hardware Status"=w175) -> (reference out=w207:refnum<vi>, error out=w213:errorcluster, 0:"error out"=w216:errorcluster)  [unwired: 7 in, 1 out]
            n77 = Merge Errors(w213, w216) -> (w206:errorcluster)
            n78 = Not A Number/Path/Refnum?(number/path/refnum=w224) -> (NaN/Path/Refnum?=w223:bool)
            n79 = property class="VI Interface Type 0"(reference=w207, error in=w206, "Exec.ShowFPOnCall"=w209, "Exec.CloseFPAfterCall"=w209) -> (reference out=w211:refnum<vi>, error out=w212:errorcluster)
            n80 = case shown="False" w223 {
              tunnel: w220 -> [w228 w229]
              tunnel: [w227 w229] -> w219
              tunnel: w217 -> [w226 _]
              tunnel: w224 -> [w225 _]
              frame False {
                n81 = property class="Str"(reference=w225, error in=w228, "Value"=w226) -> (error out=w227:errorcluster)  [unwired: 1 out]
              }
              frame True {
              }
            }
            n82 = Close Reference(reference=w211, error in (no error)=w212) -> (error out=w202:errorcluster)
            n83 = Merge Errors(w202, w219) -> (w203:errorcluster)
          }
        }
      }
      frame "Load Sequence" {
        w236 = T82 2 items=["User Home"=0, "User Desktop"=1, "User Documents"=2, "User Application Data"=3, "User Preferences"=4, "User Temporary"=5, "Public Documents"=6, "Public Application Data"=7, "Public Preferences"=8, "Public Cache"=13, "System Core Libraries"=9, "System Installed Libraries"=10, "Application Files"=11, "Boot Volume Root"=12] ("system directory type")
        n84 = call <vilib>:"Get System Directory.vi"("system directory type"=w236) -> ("system directory"=w235:path)  [unwired: 10 in]
        n85 = call "File Dialog"("start path"=w235, "prompt"="Specify the desitnation Instrument Sequence", "error in"=w256, "pattern (all files)"="*.isseq", "pattern label"="Instrument Sequence File") -> ("selected path"=w252:path, "cancelled"=w255:bool, "error out"=w254:errorcluster)  [unwired: 2 in, 6 out]
        n86 = case shown="False" w255 {
          tunnel: w254 -> [w270 w273]
          tunnel: [w265 w271] -> w243
          tunnel: w253 -> [w268 w272]
          tunnel: [w267 w272] -> w242
          tunnel: w252 -> [w266 _]
          frame False {
            n87 = Read from Binary File(5:w268, 8:w270, 11:w266) -> (0:w269:errorcluster, 2:w267:T2, 3:w264:refnum<file>)  [unwired: 1 in, 3 out]
            n88 = Close File(refnum=w264, error in=w269) -> (error out=w265:errorcluster)  [unwired: 1 out]
          }
          frame True {
            n89 = call <vilib>:"Clear Errors.vi"("error in (no error)"=w273) -> ("error out"=w271:errorcluster)  [unwired: 5 in, 1 out]
          }
        }
        n90 = Unbundle By Name(w260) -> ("Instrument Steps"=w261:refnum<vi>)
        n91 = Not A Number/Path/Refnum?(number/path/refnum=w261) -> (NaN/Path/Refnum?=w262:bool)
        n92 = case shown="False" w262 {
          tunnel: w261 -> [w275 _]
          tunnel: w242 -> [w274 _]
          frame False {
            n93 = property class="Arr (strict)"(reference=w275, "Value"=w274) -> ()  [unwired: 1 in, 2 out]
          }
          frame True {
          }
        }
        n94 = Unbundle By Name(w249) -> ("Instrument Sequence.Instrument Data"=w248:refnum<notifier>)
        n95 = Unbundle By Name(w249) -> ("Instrument Sequence.Status"=w250:refnum<notifier>)
        n96 = Unbundle By Name(w238) -> ("Plot Data"=w245:refnum<queue>)
        n97 = call "Enqueue Message (Single).vi"("error in (no error)"=w243, "Message Data"=w242, "Message"="Update Instrument Seq", "Message Queue"=w245) -> ("error out"=w241:errorcluster)  [unwired: 7 out]
        n98 = Send Notification(notification="Instrument Sequence Loaded" ("prompt"), notifier=w250, error in (no error)=w243) -> (error out=w240:errorcluster)  [unwired: 1 out]
        n99 = Send Notification(notification=w242, notifier=w248, error in (no error)=w243) -> (error out=w239:errorcluster)  [unwired: 1 out]
        n100 = Merge Errors(w241, w240, w239) -> (w246:errorcluster)
      }
      frame "Save Sequence" {
        w277 = T82 2 items=["User Home"=0, "User Desktop"=1, "User Documents"=2, "User Application Data"=3, "User Preferences"=4, "User Temporary"=5, "Public Documents"=6, "Public Application Data"=7, "Public Preferences"=8, "Public Cache"=13, "System Core Libraries"=9, "System Installed Libraries"=10, "Application Files"=11, "Boot Volume Root"=12] ("system directory type")
        n101 = call <vilib>:"Get System Directory.vi"("system directory type"=w277) -> ("system directory"=w276:path)  [unwired: 10 in]
        n102 = call "File Dialog2"("start path"=w276, "prompt"="Specify the desitnation Instrument Sequence", "error in"=w284, "pattern (all files)"="*.isseq", "pattern label"="Instrument Sequence File") -> ("selected path"=w281:path, "cancelled"=w283:bool, "error out"=w282:errorcluster)  [unwired: 2 in, 6 out]
        n103 = case shown="False" w283 {
          tunnel: w288 -> [w302 _]
          tunnel: [w294 w303] -> w278
          tunnel: w282 -> [w300 w304]
          tunnel: w281 -> [w299 _]
          tunnel: w279 -> [w295 _]
          frame False {
            n104 = Write to Binary File(file (use dialog)=w299, data=w302, error in=w300) -> (refnum out=w298:refnum<file>, error out=w301:errorcluster)  [unwired: 4 out]
            n105 = Close File(refnum=w298, error in=w301) -> (error out=w293:errorcluster)  [unwired: 1 out]
            n106 = Unbundle By Name(w295) -> ("Instrument Sequence.Status"=w296:refnum<notifier>)
            n107 = Send Notification(notification="Instrument Sequence Saved" ("prompt"), notifier=w296, error in (no error)=w293) -> (error out=w294:errorcluster)  [unwired: 1 out]
          }
          frame True {
            n108 = call <vilib>:"Clear Errors.vi"("error in (no error)"=w304) -> ("error out"=w303:errorcluster)  [unwired: 1 in, 5 out]
          }
        }
      }
      frame "Remove Step" {
        n109 = Array Size(array=w319) -> (size(s)=w321:i32)
        n110 = Decrement(x=w321) -> (x-1=w320:i32)
        n111 = Delete From Array(array=w319, length=1, index=w320) -> (array with subset deleted=w306:T2)  [unwired: 1 out]
        n112 = Unbundle By Name(w315) -> ("Instrument Sequence.Instrument Data"=w317:refnum<notifier>)
        n113 = Unbundle By Name(w315) -> ("Instrument Sequence.Status"=w316:refnum<notifier>)
        n114 = Unbundle By Name(w323) -> ("Instrument Steps"=w324:refnum<vi>)
        n115 = Unbundle By Name(w309) -> ("Plot Data"=w310:refnum<queue>)
        n116 = call "Enqueue Message (Single).vi"("error in (no error)"=w307, "Message Data"=w306, "Message"="Update Instrument Seq", "Message Queue"=w310) -> ("error out"=w308:errorcluster)  [unwired: 7 out]
        n117 = Send Notification(notification="Instrument Sequence Step Removed" ("prompt"), notifier=w316, error in (no error)=w307) -> (error out=w312:errorcluster)  [unwired: 1 out]
        n118 = Send Notification(notification=w306, notifier=w317, error in (no error)=w307) -> (error out=w313:errorcluster)  [unwired: 1 out]
        n119 = Not A Number/Path/Refnum?(number/path/refnum=w324) -> (NaN/Path/Refnum?=w325:bool)
        n120 = case shown="False" w325 {
          tunnel: w324 -> [w329 _]
          tunnel: w306 -> [w328 _]
          frame False {
            n121 = property class="Arr (strict)"(reference=w329, "Value"=w328) -> ()  [unwired: 1 in, 2 out]
          }
          frame True {
          }
        }
        n122 = Merge Errors(w308, w312, w313) -> (w314:errorcluster)
      }
      frame "Clear Sequence" {
        w336 = T2 [] ("Instrument Steps")
        n123 = Unbundle By Name(w345) -> ("Instrument Steps"=w346:refnum<vi>)
        n124 = Not A Number/Path/Refnum?(number/path/refnum=w346) -> (NaN/Path/Refnum?=w347:bool)
        n125 = case shown="False" w347 {
          tunnel: w346 -> [w353 _]
          tunnel: w336 -> [w352 _]
          tunnel: w339 -> [w351 w354]
          tunnel: [w350 w354] -> w335
          frame False {
            n126 = property class="Arr (strict)"(reference=w353, error in=w351, "Value"=w352) -> (error out=w350:errorcluster)  [unwired: 1 out]
          }
          frame True {
          }
        }
        n127 = Unbundle By Name(w341) -> ("Instrument Sequence.Instrument Data"=w343:refnum<notifier>)
        n128 = Unbundle By Name(w341) -> ("Instrument Sequence.Status"=w344:refnum<notifier>)
        n129 = Unbundle By Name(w334) -> ("Plot Data"=w337:refnum<queue>)
        n130 = call "Enqueue Message (Single).vi"("error in (no error)"=w335, "Message Data"=w336, "Message"="Update Instrument Seq", "Message Queue"=w337) -> ("error out"=w333:errorcluster)  [unwired: 7 out]
        n131 = Send Notification(notification="Instrument Sequence Cleared" ("prompt"), notifier=w344, error in (no error)=w335) -> (error out=w332:errorcluster)  [unwired: 1 out]
        n132 = Send Notification(notification=w336, notifier=w343, error in (no error)=w335) -> (error out=w331:errorcluster)  [unwired: 1 out]
        n133 = Merge Errors(w333, w332, w331) -> (w340:errorcluster)
      }
      frame "Start Sequence" {
        n134 = Unbundle By Name(w358) -> ("Instrument Sequence"=w382:refnum<queue>)
        n135 = Build Array("Update Workspace Data" ("Message"), "Reset Sequence" ("Message"), "Get Instruments Status" ("Message")) -> (w378:string[])
        n136 = call-poly "Enqueue Message.vi"("error in (no error)"=w380, "Message Array"=w378, "Message Queue"=w382) -> ("error out"=w356:errorcluster)  [unwired: 7 in, 1 out]
        n137 = Unbundle By Name(w358) -> ("Instrument Sequence"=w371:refnum<queue>)
        n138 = call-poly "Enqueue Message.vi"("error in (no error)"=w356, "Message Data"=enum16{"User", "Stress Measurement VI"}."User" ("Configuration.Caller VI"), "Message"="Measure Sequence", "Message Queue"=w371) -> ("error out"=w355:errorcluster)  [unwired: 6 in, 1 out]
        n139 = Unbundle By Name(w359) -> ("Save Data.Status"=w362:refnum<notifier>)
        n140 = Cancel Notification(0:w362, 3:w355) -> (8:w367:refnum<notifier>, 11:w365:errorcluster)  [unwired: 1 out]
        n141 = call "Wait for event.vi"("error in (no error)"=w365, "String"="Datastructures Reset", "Notifier in"=w367) -> ("error out"=w366:errorcluster)  [unwired: 7 in, 1 out]
        n142 = Unbundle By Name(w358) -> ("Save Data"=w361:refnum<queue>)
        n143 = call-poly "Enqueue Message.vi"("error in (no error)"=w365, "Message"="Set Datastructures to Default", "Message Queue"=w361) -> ("error out"=w363:errorcluster)  [unwired: 7 in, 1 out]
        n144 = Merge Errors(w363, w366) -> (w357:errorcluster)
        n145 = Unbundle By Name(w358) -> ("Plot Data"=w374:refnum<queue>)
        n146 = Build Array("Clear Sequence" ("Message"), "Disable Strain Slider" ("Message")) -> (w375:string[])
        n147 = call "Enqueue Message (Array).vi"("error in (no error)"=w357, "Message Array"=w375, "Message Queue"=w374) -> ("error out"=w372:errorcluster)  [unwired: 1 in, 7 out]
      }
      frame "Start Sequence for Strain Measurement" {
        n148 = Unbundle By Name(w391) -> ("Instrument Sequence"=w396:refnum<queue>)
        n149 = call-poly "Enqueue Message.vi"("error in (no error)"=w388, "Message"="Reset Sequence", "Message Queue"=w396) -> ("error out"=w389:errorcluster)  [unwired: 7 in, 1 out]
        n150 = Unbundle By Name(w391) -> ("Instrument Sequence"=w394:refnum<queue>)
        n151 = call-poly "Enqueue Message.vi"("error in (no error)"=w389, "Message Data"=enum16{"User", "Stress Measurement VI"}."Stress Measurement VI" ("Configuration.Caller VI"), "Message"="Measure Sequence", "Message Queue"=w394) -> ("error out"=w387:errorcluster)  [unwired: 6 in, 1 out]
      }
      frame "Measure Sequence" {
        n152 = Unbundle By Name(w406) -> ("Instrument Sequence"=w410:refnum<queue>)
        n153 = call "Enqueue Message (Single).vi"("error in (no error)"=w408, "Message"="Update Sequence Status", "Message Queue"=w410) -> ("error out"=w407:errorcluster)  [unwired: 1 in, 7 out]
        n154 = Index Array(array=w419, index=w418) -> (element=w417:T83)
        n155 = Unbundle By Name(w417) -> ("Action"=w416:T3, "Instrument"=w415:T4, "Configuration"=w414:variant)
        n156 = case shown="\"Measure\", Default" w416 {
          tunnel: w406 -> [w431 w452]
          tunnel: w415 -> [w430 w451]
          tunnel: w414 -> [_ w450]
          tunnel: [w432 w453] -> w405
          tunnel: w407 -> [w429 w449]
          frame "Measure", Default {
            n157 = case shown="\"Optoelectronic\"" w430 {
              tunnel: [w433 w438 w443 w448] -> w432
              tunnel: w431 -> [_ w437 w442 w447]
              tunnel: w429 -> [w433 w434 w439 w444]
              frame Default {
              }
              frame "Parameter Analyzer" {
                n158 = Unbundle By Name(w437) -> ("Instrument Sequence"=w436:refnum<queue>)
                n159 = call "Enqueue Message (Single).vi"("error in (no error)"=w434, "Message"="Perform Electrical Measurement", "Message Queue"=w436) -> ("error out"=w438:errorcluster)  [unwired: 1 in, 7 out]
              }
              frame "Optical Spectrometer" {
                n160 = Unbundle By Name(w442) -> ("Instrument Sequence"=w441:refnum<queue>)
                n161 = call "Enqueue Message (Single).vi"("error in (no error)"=w439, "Message"="Perform Optical Measurement", "Message Queue"=w441) -> ("error out"=w443:errorcluster)  [unwired: 1 in, 7 out]
              }
              frame "Optoelectronic" {
                n162 = Unbundle By Name(w447) -> ("Instrument Sequence"=w446:refnum<queue>)
                n163 = call "Enqueue Message (Single).vi"("error in (no error)"=w444, "Message"="Perform Optoelectronic Measurement", "Message Queue"=w446) -> ("error out"=w448:errorcluster)  [unwired: 1 in, 7 out]
              }
            }
          }
          frame "Configure" {
            n164 = case shown="\"Optical Spectrometer\"" w451 {
              tunnel: [w459 w465 w466 w472 w478] -> w453
              tunnel: w452 -> [w458 w464 _ w471 w477]
              tunnel: w450 -> [w455 w461 _ w468 w474]
              tunnel: w449 -> [w454 w462 w466 w467 w473]
              frame "Parameter Analyzer" {
                n165 = Unbundle By Name(w458) -> ("Instrument Sequence"=w457:refnum<queue>)
                n166 = call "Enqueue Message (Single).vi"("error in (no error)"=w454, "Message Data"=w455, "Message"="Configure Parameter Analyzer", "Message Queue"=w457) -> ("error out"=w459:errorcluster)  [unwired: 7 out]
              }
              frame "Autofocus" {
                n167 = Unbundle By Name(w464) -> ("Instrument Sequence"=w463:refnum<queue>)
                n168 = call-poly "Enqueue Message.vi"("error in (no error)"=w462, "Message Data"=w461, "Message"="Focus", "Message Queue"=w463) -> ("error out"=w465:errorcluster)  [unwired: 6 in, 1 out]
              }
              frame "Unknown Instrument", Default {
              }
              frame "Switching Matrix" {
                n169 = Unbundle By Name(w471) -> ("Instrument Sequence"=w470:refnum<queue>)
                n170 = call "Enqueue Message (Single).vi"("error in (no error)"=w467, "Message Data"=w468, "Message"="Configure Switching Matrix", "Message Queue"=w470) -> ("error out"=w472:errorcluster)  [unwired: 7 out]
              }
              frame "Optical Spectrometer" {
                n171 = Unbundle By Name(w477) -> ("Instrument Sequence"=w476:refnum<queue>)
                n172 = call "Enqueue Message (Single).vi"("error in (no error)"=w473, "Message Data"=w474, "Message"="Configure Optical Spectrometer", "Message Queue"=w476) -> ("error out"=w478:errorcluster)  [unwired: 7 out]
              }
            }
          }
        }
        n173 = case shown="\"User\", Default" w402 {
          tunnel: w406 -> [w426 _]
          tunnel: w405 -> [w424 w428]
          tunnel: [w423 w428] -> w404
          frame "User", Default {
            n174 = Unbundle By Name(w426) -> ("Instrument Sequence"=w427:refnum<queue>)
            n175 = call "Enqueue Message (Single).vi"("error in (no error)"=w424, "Message"="Save Measured Sequence", "Message Queue"=w427) -> ("error out"=w423:errorcluster)  [unwired: 1 in, 7 out]
          }
          frame "Stress Measurement VI" {
          }
        }
        n176 = Unbundle By Name(w406) -> ("Instrument Sequence"=w413:refnum<queue>)
        n177 = call "Enqueue Message (Single).vi"("error in (no error)"=w404, "Message Data"=w402, "Message"="Choose What Next", "Message Queue"=w413) -> ("error out"=w411:errorcluster)  [unwired: 7 out]
      }
      frame "Reset Sequence" {
        n178 = for {
          tunnel: w495 -> [w504] mode=indexing
          tunnel: [w502] -> w482 mode=indexing
          n179 = Bundle By Name(cluster=w504, "Status"=enum8{"False", "True", "Mixed"}."False") -> (w502:T83)
        }
        n180 = Unbundle By Name(w483) -> ("Instrument Steps"=w484:refnum<vi>)
        n181 = Not A Number/Path/Refnum?(number/path/refnum=w484) -> (NaN/Path/Refnum?=w485:bool)
        n182 = case shown="False" w485 {
          tunnel: w484 -> [w500 _]
          tunnel: w481 -> [w499 w501]
          tunnel: [w498 w501] -> w480
          tunnel: w482 -> [w497 _]
          frame False {
            n183 = property class="Arr (strict)"(reference=w500, error in=w499, "Value"=w497) -> (error out=w498:errorcluster)  [unwired: 1 out]
          }
          frame True {
          }
        }
        n184 = Unbundle By Name(w486) -> ("Instrument Sequence.Instrument Data"=w489:refnum<notifier>)
        n185 = Unbundle By Name(w486) -> ("Instrument Sequence.Status"=w488:refnum<notifier>)
        n186 = Send Notification(notification="Instrument Sequence Reset" ("prompt"), notifier=w488, error in (no error)=w480) -> (error out=w492:errorcluster)  [unwired: 1 out]
        n187 = Send Notification(notification=w482, notifier=w489, error in (no error)=w480) -> (error out=w491:errorcluster)  [unwired: 1 out]
        n188 = Merge Errors(w492, w491) -> (w487:errorcluster)
      }
      frame "Update Sequence Status" {
        # "Current Index within array size"
        n189 = Greater Than 0?(x=w509) -> (x > 0?=w523:bool)
        n190 = Index Array(array=w510, index=w509) -> (element=w508:T83)
        n191 = Bundle By Name(cluster=w508, "Status"=enum8{"False", "True", "Mixed"}."Mixed") -> (w506:T83)
        n192 = Replace Array Subset(array=w510, new element=w506, index=w509) -> (w524:T2)
        n193 = case shown="True" w523 {
          tunnel: w509 -> [_ w536]
          tunnel: w524 -> [w532 w535]
          tunnel: [w532 w533] -> w511
          frame False {
            # "There are no previous points"
          }
          frame True {
            # "Set that Previous Point has been measured"
            n194 = Decrement(x=w536) -> (x-1=w534:i32)
            n195 = Index Array(array=w535, index=w534) -> (element=w537:T83)
            n196 = Bundle By Name(cluster=w537, "Status"=enum8{"False", "True", "Mixed"}."True") -> (w539:T83)
            n197 = Replace Array Subset(array=w535, new element=w539, index=w534) -> (w533:T2)
          }
        }
        n198 = Unbundle By Name(w522) -> ("Instrument Steps"=w520:refnum<vi>)
        n199 = Not A Number/Path/Refnum?(number/path/refnum=w520) -> (NaN/Path/Refnum?=w521:bool)
        n200 = case shown="False" w521 {
          tunnel: w520 -> [w530 _]
          tunnel: w511 -> [w529 _]
          tunnel: w519 -> [w528 w531]
          tunnel: [w527 w531] -> w513
          frame False {
            n201 = property class="Arr (strict)"(reference=w530, error in=w528, "Value"=w529) -> (error out=w527:errorcluster)  [unwired: 1 out]
          }
          frame True {
          }
        }
        n202 = Unbundle By Name(w512) -> ("Instrument Sequence.Instrument Data"=w517:refnum<notifier>)
        n203 = Unbundle By Name(w512) -> ("Instrument Sequence.Status"=w518:refnum<notifier>)
        n204 = Send Notification(notification="Instrument Sequence Updated" ("prompt"), notifier=w518, error in (no error)=w513) -> (error out=w514:errorcluster)  [unwired: 1 out]
        n205 = Send Notification(notification=w511, notifier=w517, error in (no error)=w513) -> (error out=w515:errorcluster)  [unwired: 1 out]
        n206 = Merge Errors(w514, w515) -> ()  [unwired: 1 out]
      }
      frame "Choose What Next" {
        n207 = Array Size(array=w545) -> (size(s)=w549:i32)
        n208 = Decrement(x=w549) -> (x-1=w553:i32)
        n209 = Less?(x=w548, y=w553) -> (x < y?=w552:bool)
        n210 = case shown="True" w552 {
          tunnel: w550 -> [w561 w564]
          tunnel: [w555 w569] -> w551
          tunnel: [w560 w574] -> w547
          tunnel: w548 -> [w558 w573]
          tunnel: w542 -> [_ w572]
          tunnel: w544 -> [w556 w570]
          tunnel: w543 -> [w554 w571]
          tunnel: w540 -> [_ w562]
          frame True {
            # "There's at least \none more datapoint"
            n211 = Unbundle By Name(w556) -> ("Instrument Sequence"=w557:refnum<queue>)
            n212 = Increment(x=w558) -> (x+1=w560:i32)
            n213 = call "Enqueue Message (Single).vi"("error in (no error)"=w561, "Message Data"=w554, "Message"="Measure Sequence", "Message Queue"=w557) -> ("error out"=w555:errorcluster)  [unwired: 7 out]
          }
          frame False {
            n214 = case shown="\"User\", Default" w571 {
              tunnel: w564 -> [w581 w586]
              tunnel: w570 -> [w583 _]
              tunnel: [w575 w586] -> w563
              tunnel: w572 -> [w582 _]
              tunnel: w562 -> [w578 _]
              frame "User", Default {
                n215 = Unbundle By Name(w578) -> ("Save Data.Status"=w577:refnum<notifier>)
                n216 = Cancel Notification(0:w577, 3:w581) -> (11:w580:errorcluster)  [unwired: 2 out]
                n217 = Unbundle By Name(w583) -> ("Save Data"=w585:refnum<queue>)
                n218 = call "Enqueue Message (Single).vi"("error in (no error)"=w580, "Message Data"=w582, "Message"="Pickle2Workspace", "Message Queue"=w585) -> ("error out"=w576:errorcluster)  [unwired: 7 out]
                n219 = call "Wait for event.vi"("error in (no error)"=w576, "String"="Workspace file saved", "Notifier in"=w577) -> ("error out"=w575:errorcluster)  [unwired: 7 in, 1 out]
              }
              frame "Stress Measurement VI" {
              }
            }
            n220 = Unbundle By Name(w570) -> ("Instrument Sequence"=w568:refnum<queue>)
            n221 = Increment(x=w573) -> (x+1=w574:i32)
            n222 = Build Array("Update Sequence Status" ("Message"), "Declare Completion" ("Message")) -> (w567:string[])
            n223 = call "Enqueue Message (Array).vi"("error in (no error)"=w563, "Message Array"=w567, "Message Queue"=w568) -> ("error out"=w569:errorcluster)  [unwired: 1 in, 7 out]
          }
        }
      }
      frame "Update Workspace Data" {
        n224 = call "Set Device Information.vi"() -> ("error out"=w595:errorcluster, "Workspace Info"=w588:T84, "OK?"=w591:bool)  [unwired: 9 out]
        n225 = Merge Errors(w595, w597) -> (w596:errorcluster)
        n226 = case shown="True" w591 {
          tunnel: w596 -> [w601 w615]
          tunnel: w588 -> [_ w614]
          tunnel: w594 -> [_ w613]
          tunnel: [w600 w611] -> w593
          tunnel: w590 -> [w602 _]
          frame False {
            n227 = Unbundle By Name(w602) -> ("Instrument Sequence"=w604:refnum<queue>)
            n228 = call "Enqueue Message (Single).vi"("Priority Message? (F)"=TRUE, "error in (no error)"=w601, "Message"="Stop Sequence", "Message Queue"=w604) -> ("error out"=w600:errorcluster)  [unwired: 1 in, 6 out]
          }
          frame True {
            n229 = Unbundle By Name(w613) -> ("Device ID"=w607:refnum<vi>, "Device Information"=w605:refnum<vi>)
            n230 = Unbundle By Name(w614) -> ("Device Name"=w609:string, "Device Info"=w610:string)
            "Device Name" <- w609
            "Device Info" <- w610
            n231 = Not A Number/Path/Refnum?(number/path/refnum=w607) -> (NaN/Path/Refnum?=w608:bool)
            n232 = case shown="False" w608 {
              tunnel: w615 -> [w624 w625]
              tunnel: [w623 w625] -> w612
              tunnel: w609 -> [w622 _]
              tunnel: w607 -> [w621 _]
              frame False {
                n233 = property class="Str"(reference=w621, error in=w624, "Value"=w622) -> (error out=w623:errorcluster)  [unwired: 1 out]
              }
              frame True {
              }
            }
            n234 = Not A Number/Path/Refnum?(number/path/refnum=w605) -> (NaN/Path/Refnum?=w606:bool)
            n235 = case shown="False" w606 {
              tunnel: w612 -> [w619 w620]
              tunnel: [w618 w620] -> w611
              tunnel: w610 -> [w617 _]
              tunnel: w605 -> [w616 _]
              frame False {
                n236 = property class="Str"(reference=w616, error in=w619, "Value"=w617) -> (error out=w618:errorcluster)  [unwired: 1 out]
              }
              frame True {
              }
            }
          }
        }
      }
      frame "Save Measured Sequence" {
        n237 = Unbundle By Name(w633) -> ("Save Data.Status"=w632:refnum<notifier>)
        n238 = Cancel Notification(0:w632, 3:w631) -> (8:w630:refnum<notifier>, 11:w629:errorcluster)  [unwired: 1 out]
        n239 = Unbundle By Name(w642) -> ("Save Data"=w637:refnum<queue>)
        n240 = call "Enqueue Message (Single).vi"("error in (no error)"=w629, "Message Data"=w635, "Message"="Save Measured Sequence", "Message Queue"=w637) -> ("error out"=w626:errorcluster)  [unwired: 7 out]
        n241 = call "Wait for event.vi"("error in (no error)"=w629, "String"="Instrument Sequence Saved", "Notifier in"=w630) -> ("error out"=w628:errorcluster)  [unwired: 7 in, 1 out]
        n242 = Merge Errors(w626, w628) -> (w627:errorcluster)
      }
      frame "Get Instruments Status" {
        w645 = T60 {"Parameter Analyzer"={"Configuration"={"Parameter Analyzer VISA Session"="COM1", "Sweeping Time Parameters"={"Integration Time"=0, "Short Integration Time (s)"=1.0, "Long Integration Time (s)"=0.0, "Wait Time Parameter"=1.0}, "Acquisition Mode"=enum."Sweeping Mode", "Status Polling Time (ms)"=1000, "Comment"="Test VI", "SMU 1 - Sweeping"={"Start / Offset"=0.0, "Stop / Ratio"=1.0, "Step \n(linear only)"=0.01, "Compliance"=0.1, "Power \nCompliance"=0.0, "Mode"=0, "Function"=0, "Sweep Mode"=FALSE}, "SMU 2 - Sweeping"={"Start / Offset"=0.0, "Stop / Ratio"=1.0, "Step \n(linear only)"=0.01, "Compliance"=0.1, "Power \nCompliance"=0.0, "Mode"=0, "Function"=0, "Sweep Mode"=FALSE}, "SMU 3 - Sweeping"={"Start / Offset"=0.0, "Stop / Ratio"=1.0, "Step \n(linear only)"=0.01, "Compliance"=0.1, "Power \nCompliance"=0.0, "Mode"=0, "Function"=0, "Sweep Mode"=FALSE}, "SMU 4 - Sweeping"={"Start / Offset"=0.0, "Stop / Ratio"=1.0, "Step \n(linear only)"=0.01, "Compliance"=0.1, "Power \nCompliance"=0.0, "Mode"=0, "Function"=0, "Sweep Mode"=FALSE}, "Sweep Spacing"=0, "Range"=0, "SMU1 - Sampling"={"Source"=10.0, "Compliance"=1e-05, "Mode"=0, "Function"=FALSE}, "SMU2 - Sampling"={"Source"=10.0, "Compliance"=1e-05, "Mode"=0, "Function"=FALSE}, "SMU3 - Sampling"={"Source"=10.0, "Compliance"=1e-05, "Mode"=0, "Function"=FALSE}, "SMU4 - Sampling"={"Source"=0.1, "Compliance"=60.0, "Mode"=10, "Function"=FALSE}, "Sampling Time Parameters"={"Initial Interval (s)"=0.1, "Number of Samples"=60, "Total Sampling Time (s)"=10.0, "Hold Time (s)"=0.0, "Sampling Mode"=0, "Sampling Time"=0}, "Stop Condition"={"Enable Delay (s)"=0.0, "Name"="", "Threshold"=0.0, "num. of events"=1, "Event"=0, "Stop Condition Enable"=FALSE}}, "Refnums"={"Status"=refnum, "Electrical Measurement"=refnum, "Plots"={"Plot List"=refnum, "Voltage Plot"=refnum, "Current Plot"=refnum, "IV Characteristic"=refnum, "dI/dV-V Characteristic"=refnum}, "HP Integration Time"=refnum, "VISA"=refnum, "Sweeping Time Parameters"=refnum, "Acquisition Mode"=refnum, "SMU 1 - Sweeping"=refnum, "SMU 2 - Sweeping"=refnum, "SMU 3 - Sweeping"=refnum, "SMU 4 - Sweeping"=refnum, "Sweep Spacing"=refnum, "Range"=refnum, "SMU1 - Sampling"=refnum, "SMU2 - Sampling"=refnum, "SMU3 - Sampling"=refnum, "SMU4 - Sampling"=refnum, "Sampling Time Parameters"=refnum, "Stop Condition"=refnum, "Instrument Status"=refnum}, "Initialization"={"Update Visa Session"=FALSE, "Configure Integration Time"=FALSE, "Configure Acquisition Mode"=FALSE, "Update Refnums"=FALSE}}, "Swithing Matrix"={"Configuration"={"Switching Matrix VISA Session"="GPIB0::18::INSTR", "Connections"=[{"Connections"=[FALSE, FALSE, FALSE, FALSE, FALSE, FALSE, FALSE, FALSE, FALSE, FALSE, FALSE, FALSE], "Connection Type"=enum."Disconnected"}, {"Connections"=[FALSE, FALSE, FALSE, FALSE, FALSE, FALSE, FALSE, FALSE, FALSE, FALSE, FALSE, FALSE], "Connection Type"=enum."Disconnected"}, {"Connections"=[FALSE, FALSE, FALSE, FALSE, FALSE, FALSE, FALSE, FALSE, FALSE, FALSE, FALSE, FALSE], "Connection Type"=enum."Disconnected"}, {"Connections"=[FALSE, FALSE, FALSE, FALSE, FALSE, FALSE, FALSE, FALSE, FALSE, FALSE, FALSE, FALSE], "Connection Type"=enum."Disconnected"}, {"Connections"=[FALSE, FALSE, FALSE, FALSE, FALSE, FALSE, FALSE, FALSE, FALSE, FALSE, FALSE, FALSE], "Connection Type"=enum."Disconnected"}, {"Connections"=[FALSE, FALSE, FALSE, FALSE, FALSE, FALSE, FALSE, FALSE, FALSE, FALSE, FALSE, FALSE], "Connection Type"=enum."Disconnected"}, {"Connections"=[FALSE, FALSE, FALSE, FALSE, FALSE, FALSE, FALSE, FALSE, FALSE, FALSE, FALSE, FALSE], "Connection Type"=enum."Disconnected"}, {"Connections"=[FALSE, FALSE, FALSE, FALSE, FALSE, FALSE, FALSE, FALSE, FALSE, FALSE, FALSE, FALSE], "Connection Type"=enum."Disconnected"}]}, "Refnums"={"Connections"=refnum, "Instrument Status"=refnum}, "Initialization"={"Update Visa Session"=FALSE, "Update Refnums"=FALSE}}, "Stress Control"={"Configuration"={"Stress Control VISA Session"="StrainMotor", "Axis"=0, "Motion"=0, "Destination (°)"=0.0, "Speed (°/s)"=4.0, "Position (°)"=25.0}, "Refnums"={"Instrument Status"=refnum, "Position"=refnum, "Mecahnism Motion"=refnum, "Destination"=refnum, "Apply Stress"=refnum, "Stop"=refnum, "Stress Control VISA"=refnum}, "Initialization"={"Update Visa Session"=FALSE, "Update Configuration"=FALSE, "Update Refnums"=FALSE, "Get Position"=FALSE}}, "Optical Spectrometer"={"Configuration"={"Laser Settings"={"Laser Wavelength"=enum."784 nm", "Neutral Density Filter"=enum."50%"}, "Spectrometer Settings"={"Confocal Hole Size (µm)"=150.0, "Grating"=2, "Detector"=enum."InGaAs Array"}, "Acquisition Settings"={"Acquisition Mode"=enum."Multi-Window", "Spectal Position (nm)"=632.0, "From (nm)"=735.0, "To (nm)"=3.0, "Integration Time (s)"=3.0, "Number of Accumulations"=3, "AutoScanning"=FALSE, "Spike Removal"=FALSE}, "Path"=path "C:/07 - Prizes and Awards/Marie Curie Prize/Reply Editors Final NCOMMS(10).docx"}, "Refnums"={"Instrument Status"=refnum, "Optical Spectrum Plot"={"Plot List"=refnum, "Optical Spectrum vs Energy"=refnum, "Optical Spectrum vs Wavelength"=refnum, "Optical Spectrum vs Raman Shift"=refnum, "Detector Temperature"=refnum}, "Laser"=refnum, "Filter"=refnum, "Laser ON?"=refnum, "Hole"=refnum, "Grating"=refnum, "Detector"=refnum, "Acquisition Mode"=refnum, "Spectal Position"=refnum, "From"=refnum, "To"=refnum, "Integration Time"=refnum, "Accumulations"=refnum, "AutoScanning"=refnum, "Spike Removal"=refnum, "Acquisition Mode Panel"=refnum}, "Initialization"={"Connect"=FALSE, "Update Refnums"=FALSE, "Get Configuration"=FALSE}}, "Switches & Mirrors"={"Configuration"={"Relay VISA Session"="COM1", "Switches"={"Laser"=FALSE, "Video"=FALSE}, "Delays (ms)"={"Laser"=500, "Video"=1500}}, "Refnums"={"Instrument Status"=refnum, "Laser"=refnum, "Video"=refnum, "Relay VISA"=refnum}, "Initialize"={"Update Refnums"=FALSE, "Connect"=FALSE, "Set Configuration"=FALSE}}, "Camera"={"Configuration"={"Settings"={"Pixel clock"=20, "Frame rate"=30.0, "Exposure time"=33.21525, "Master Gain"=0, "Red Gain"=0, "Green Gain"=0, "Blue Gain"=0, "Auto Gain"=FALSE, "White-balance"=FALSE, "Color Correction"=FALSE}}, "Refnums"={"Pixel Clock"=refnum, "Frame Rate"=refnum, "Exposure Time"=refnum, "Master Gain"=refnum, "Red Gain"=refnum, "Green Gain"=refnum, "Blue Gain"=refnum, "Auto Gain"=refnum, "Auto White-balance"=refnum, "Color Correction"=refnum, "Image"=refnum, "Video Button"=refnum, "Instrument Status"=refnum}, "Initialization"={"Connect"=FALSE, "Update Refnums"=FALSE, "Acquiring?"=FALSE}}, "XYZ Stage"={"Configuration"={"Connection Settings"={"Tango VISA"="", "Baudrate"=57600, "Show Protocol?"=FALSE}, "Manual Control"={"North"=FALSE, "South"=FALSE, "West"=FALSE, "East"=FALSE, "Up"=FALSE, "Down"=FALSE, "Stop"=FALSE, "XY Step"=0.0, "Z step"=0.0}, "Coordinate Control"={"Motion Mode"=enum."Absolute", "Destination [mm]"=[]}}, "Refnums"={"Instrument Status"=refnum, "Position"=refnum, "Manual Control"=refnum, "Up"=refnum, "Down"=refnum, "North"=refnum, "South"=refnum, "East"=refnum, "West"=refnum, "Stop"=refnum, "Limits"=refnum}, "Initialization"={"Update Visa Session"=FALSE, "Set To Default"=FALSE, "Get Status"=FALSE, "Update Refnums"=FALSE}}, "AutoFocus"={"Configuration"={"Matching Criteria"={"Minimum Score"=700.0, "Color Score Weight"=700.0, "Minimum Contrast"=50, "Match Mode"=0, "Match Feature Mode"=0, "Subpixel Accuracy"=TRUE, "Color Sensitivity"=1, "Search Strategy"=1}, "Z Scan Parameters"={"Z Range"=1380.0, "Resolution"=5000.0, "Initial Direction"=enum."Up", "Focus Threshold"=0.1, "Ascent Constant"=0.1}, "Displacement"=0.0, "Transformation Matrix"=[]}, "Refnums"={"Instrument Status"=refnum, "Matching Criteria"=refnum, "Z Scan Parameters"=refnum, "Distance"=refnum, "Transformation Matrix"=refnum, "Match and Edge"={"Image"=refnum, "Target"=refnum, "Edge"=refnum, "Target Data"=refnum}, "Matching Curves"=refnum, "Tracking"=refnum, "Focus"=refnum, "Find Focus"=refnum, "Set Target"=refnum, "Link Stage & Camera"=refnum, "Align"=refnum}, "Initialize"={"Update Refnums"=FALSE, "Allocate Image Memory"=FALSE, "Set Match Criteria"=FALSE, "Link Stage & Camera"=FALSE, "Set Target"=FALSE, "Find Target"=FALSE}}} ("Instruments Status")
        n243 = Unbundle By Name(w659) -> ("Parameter Analyzer.Instrument Data"=w654:refnum<notifier>, "Switching Matrix.Instrument Data"=w653:refnum<notifier>, "Optical Spectrometer.Instrument Data"=w650:refnum<notifier>, "AutoFocus.Instrument Data"=w647:refnum<notifier>)
        n244 = Unbundle By Name(w645) -> ("Parameter Analyzer"=w656:T26, "Swithing Matrix"=w655:T37, "Optical Spectrometer"=w649:T41, "AutoFocus"=w646:T53)
        n245 = case shown="\"Full Instrument Palette\", Default" w643 {
          tunnel: [w704 w731] -> w661
          tunnel: w658 -> [w703 w730]
          tunnel: [w697 w725] -> w657
          tunnel: w656 -> [w696 w724]
          tunnel: w655 -> [w695 w723]
          tunnel: w654 -> [w693 w721]
          tunnel: w653 -> [w692 w720]
          tunnel: w650 -> [w681 _]
          tunnel: w649 -> [w680 _]
          tunnel: w648 -> [w677 w712]
          tunnel: w647 -> [w675 _]
          tunnel: w646 -> [w672 _]
          tunnel: w645 -> [w663 w707]
          frame "Full Instrument Palette", Default {
            w665 = "Notify Status" ("Message")
            n246 = Cancel Notification(0:w681, 3:w677) -> (11:w685:errorcluster)  [unwired: 2 out]
            n247 = Cancel Notification(0:w692, 3:w677) -> (11:w691:errorcluster)  [unwired: 2 out]
            n248 = Cancel Notification(0:w675, 3:w677) -> (11:w676:errorcluster)  [unwired: 2 out]
            n249 = Cancel Notification(0:w693, 3:w677) -> (11:w690:errorcluster)  [unwired: 2 out]
            n250 = Merge Errors(w690, w691, w685, w676) -> (w666:errorcluster)
            n251 = Unbundle By Name(w703) -> ("Optical Spectrometer"=w670:refnum<queue>, "Parameter Analyzer"=w669:refnum<queue>, "Switching Matrix"=w668:refnum<queue>, "AutoFocus"=w667:refnum<queue>)
            n252 = Wait on Notification(notifier=w692, error in (no error)=w666) -> (notification=w698:variant, error out=w699:errorcluster)  [unwired: 4 out]
            n253 = Wait on Notification(notifier=w693, error in (no error)=w666) -> (notification=w706:variant, error out=w705:errorcluster)  [unwired: 4 out]
            n254 = Wait on Notification(notifier=w681, error in (no error)=w666) -> (notification=w682:variant, error out=w684:errorcluster)  [unwired: 4 out]
            n255 = Wait on Notification(notifier=w675, error in (no error)=w666) -> (notification=w674:variant, error out=w673:errorcluster)  [unwired: 4 out]
            n256 = call "Enqueue Message (Single).vi"("error in (no error)"=w666, "Message"=w665, "Message Queue"=w670) -> ("error out"=w664:errorcluster)  [unwired: 1 in, 7 out]
            n257 = call "Enqueue Message (Single).vi"("error in (no error)"=w666, "Message"=w665, "Message Queue"=w668) -> ("error out"=w701:errorcluster)  [unwired: 1 in, 7 out]
            n258 = call "Enqueue Message (Single).vi"("error in (no error)"=w666, "Message"=w665, "Message Queue"=w669) -> ("error out"=w702:errorcluster)  [unwired: 1 in, 7 out]
            n259 = call "Enqueue Message (Single).vi"("error in (no error)"=w666, "Message"=w665, "Message Queue"=w667) -> ("error out"=w700:errorcluster)  [unwired: 1 in, 7 out]
            n260 = Variant To Data(error in=w699, type=w695, Variant=w698) -> (data=w678:T37, error out=w688:errorcluster)
            n261 = Variant To Data(error in=w684, type=w680, Variant=w682) -> (data=w679:T41, error out=w683:errorcluster)
            n262 = Variant To Data(error in=w673, type=w672, Variant=w674) -> (data=w662:T53, error out=w671:errorcluster)
            n263 = Variant To Data(error in=w705, type=w696, Variant=w706) -> (data=w694:T26, error out=w689:errorcluster)
            n264 = Bundle By Name(cluster=w663, "Parameter Analyzer"=w694, "Swithing Matrix"=w678, "Optical Spectrometer"=w679, "AutoFocus"=w662) -> (w697:T60)
            n265 = Merge Errors(w689, w688, w683, w671) -> (w687:errorcluster)
            n266 = Merge Errors(w664, w702, w701, w700) -> (w686:errorcluster)
            n267 = Merge Errors(w687, w686) -> (w704:errorcluster)
          }
          frame "Strain Electrical" {
            w708 = "Notify Status" ("Message")
            n268 = Cancel Notification(0:w720, 3:w712) -> (11:w719:errorcluster)  [unwired: 2 out]
            n269 = Cancel Notification(0:w721, 3:w712) -> (11:w718:errorcluster)  [unwired: 2 out]
            n270 = Merge Errors(w718, w719) -> (w709:errorcluster)
            n271 = Unbundle By Name(w730) -> ("Parameter Analyzer"=w711:refnum<queue>, "Switching Matrix"=w710:refnum<queue>)
            n272 = Wait on Notification(notifier=w720, error in (no error)=w709) -> (notification=w726:variant, error out=w727:errorcluster)  [unwired: 4 out]
            n273 = Wait on Notification(notifier=w721, error in (no error)=w709) -> (notification=w733:variant, error out=w732:errorcluster)  [unwired: 4 out]
            n274 = call "Enqueue Message (Single).vi"("error in (no error)"=w709, "Message"=w708, "Message Queue"=w710) -> ("error out"=w728:errorcluster)  [unwired: 1 in, 7 out]
            n275 = call "Enqueue Message (Single).vi"("error in (no error)"=w709, "Message"=w708, "Message Queue"=w711) -> ("error out"=w729:errorcluster)  [unwired: 1 in, 7 out]
            n276 = Variant To Data(error in=w727, type=w723, Variant=w726) -> (data=w713:T37, error out=w716:errorcluster)
            n277 = Variant To Data(error in=w732, type=w724, Variant=w733) -> (data=w722:T26, error out=w717:errorcluster)
            n278 = Bundle By Name(cluster=w707, "Parameter Analyzer"=w722, "Swithing Matrix"=w713) -> (w725:T60)
            n279 = Merge Errors(w717, w716) -> (w715:errorcluster)
            n280 = Merge Errors(w729, w728) -> (w714:errorcluster)
            n281 = Merge Errors(w715, w714) -> (w731:errorcluster)
          }
        }
      }
      frame "Get Autofocus Status" {
        n282 = Unbundle By Name(w754) -> ("AutoFocus.Instrument Data"=w748:refnum<notifier>)
        n283 = Cancel Notification(0:w748, 3:w749) -> (8:w739:refnum<notifier>, 11:w735:errorcluster)  [unwired: 1 out]
        n284 = Unbundle By Name(w753) -> ("AutoFocus"=w745:refnum<queue>)
        n285 = Wait on Notification(notifier=w739, error in (no error)=w735) -> (notification=w747:variant, error out=w736:errorcluster)  [unwired: 4 out]
        n286 = call "Enqueue Message (Single).vi"("error in (no error)"=w735, "Message"="Notify Status", "Message Queue"=w745) -> ("error out"=w740:errorcluster)  [unwired: 1 in, 7 out]
        n287 = Merge Errors(w740, w736) -> (w737:errorcluster)
        n288 = Unbundle By Name(w741) -> ("AutoFocus"=w746:T53)
        n289 = Variant To Data(error in=w737, type=w746, Variant=w747) -> (data=w743:T53, error out=w738:errorcluster)
        n290 = Unbundle By Name(w743) -> ("Initialize"=w734:T59)
        n291 = Bundle By Name(cluster=w741, "AutoFocus.Initialize"=w734) -> (w752:T60)
      }
      frame "Perform Electrical Measurement" {
        # "Data Saved in \nWorkspace by \nHP.vi already"
        n292 = Unbundle By Name(w790) -> ("Save Data.Status"=w764:refnum<notifier>, "Parameter Analyzer.Measurement"=w799:refnum<notifier>)
        n293 = Unbundle By Name(w778) -> ("Parameter Analyzer.Configuration.Acquisition Mode"=w780:enum32{"Sweeping Mode", "Sampling Mode"})
        n294 = Cancel Notification(0:w799, 3:w763) -> (8:w803:refnum<notifier>, 11:w758:errorcluster)  [unwired: 1 out]
        n295 = Wait on Notification(notifier=w803, error in (no error)=w758) -> (notification=w801:variant, error out=w800:errorcluster)  [unwired: 4 out]
        n296 = Variant To Data(error in=w800, type=T23 {"Sequence"=[], "V1"=[], "V2"=[], "V3"=[], "V4"=[], "I1"=[], "I2"=[], "I3"=[], "I4"=[]} ("Measurement"), Variant=w801) -> (data=w781:T23, error out=w757:errorcluster)
        n297 = call "Measurement.vi"() -> ("Measurement"=w779:T85)
        n298 = Bundle By Name(cluster=w779, "Electrical Measurement"=w781, "Which Instrument?"=WhichInstrument."Parameter Analyzer", "Measurement Mode"=w780) -> (w783:T85)
        n299 = Cancel Notification(0:w764, 3:w757) -> (11:w756:errorcluster)  [unwired: 2 out]
        n300 = Unbundle By Name(w790) -> ("Save Data.Status"=w773:refnum<notifier>)
        n301 = Unbundle By Name(w765) -> ("Plot Data"=w785:refnum<queue>)
        n302 = Unbundle By Name(w790) -> ("Instrument Sequence.Measurement"=w791:refnum<notifier>)
        n303 = Unbundle By Name(w790) -> ("Instrument Sequence.Status"=w793:refnum<notifier>)
        n304 = Unbundle By Name(w778) -> ("Parameter Analyzer.Configuration"=w777:T27)
        n305 = call "Enqueue Message (Single).vi"("error in (no error)"=w756, "Message Data"=w783, "Message"="Append Measurement", "Message Queue"=w785) -> ("error out"=w784:errorcluster)  [unwired: 7 out]
        n306 = call "Wait for event.vi"("error in (no error)"=w756, "String"="Electrical Data Updated", "Notifier in"=w773) -> ("error out"=w762:errorcluster, "Notifier out"=w761:refnum<notifier>)  [unwired: 7 in]
        n307 = Cancel Notification(0:w761, 3:w762) -> (8:w760:refnum<notifier>, 11:w759:errorcluster)  [unwired: 1 out]
        n308 = Send Notification(notification="Electrical Measurement Performed" ("Message"), notifier=w793, error in (no error)=w756) -> (error out=w787:errorcluster)  [unwired: 1 out]
        n309 = Send Notification(notification=w781, notifier=w791, error in (no error)=w756) -> (error out=w788:errorcluster)  [unwired: 1 out]
        n310 = Unbundle By Name(w765) -> ("Parameter Analyzer"=w797:refnum<queue>)
        n311 = call "Enqueue Message (Single).vi"("error in (no error)"=w758, "Message Data"=w777, "Message"="Measure", "Message Queue"=w797) -> ("error out"=w789:errorcluster)  [unwired: 7 out]
        n312 = Unbundle By Name(w765) -> ("Save Data"=w768:refnum<queue>)
        n313 = Build Array("Append Electrical Data" ("Message"), "Append Instrument Sequence Step" ("Message")) -> (w769:string[])
        n314 = call "Wait for event.vi"("error in (no error)"=w759, "String"="Instrument Sequence Step Appended", "Notifier in"=w760) -> ("error out"=w767:errorcluster)  [unwired: 7 in, 1 out]
        n315 = call "Enqueue Message (Array).vi"("error in (no error)"=w759, "Message Array"=w769, "Message Queue"=w768) -> ("error out"=w766:errorcluster)  [unwired: 7 in, 1 out]
        n316 = Merge Errors(w789, w787, w788, w766, w767, w784) -> (w776:errorcluster)
      }
      frame "Perform Optical Measurement" {
        w830 = T66 {"Relay VISA Session"="COM1", "Switches"={"Laser"=FALSE, "Video"=FALSE}, "Delays (ms)"={"Laser"=500, "Video"=1500}}  # Video Off
        w840 = T66 {"Relay VISA Session"="COM1", "Switches"={"Laser"=FALSE, "Video"=FALSE}, "Delays (ms)"={"Laser"=500, "Video"=1500}}  # Laser Off
        # "Data Saved in \nWorkspace by \nTool already"
        n317 = Unbundle By Name(w805) -> ("Switches & Mirrors.Configuration.Switches.Laser"=w828:bool)
        n318 = Unbundle By Name(w832) -> ("Save Data.Status"=w809:refnum<notifier>, "Optical Spectrometer.Measurement"=w808:refnum<notifier>, "Switches & Mirrors.Status"=w843:refnum<notifier>)
        n319 = Cancel Notification(0:w843, 3:w816) -> (8:w827:refnum<notifier>, 11:w812:errorcluster)  [unwired: 1 out]
        n320 = Unbundle By Name(w834) -> ("Switches & Mirrors"=w845:refnum<queue>)
        n321 = Bundle By Name(cluster=w830, "Switches.Laser"=w828) -> (w829:T66)
        n322 = call "Wait for event.vi"("error in (no error)"=w812, "String"="Configuration Set", "Notifier in"=w827) -> ("error out"=w826:errorcluster)  [unwired: 7 in, 1 out]
        n323 = call "Enqueue Message (Single).vi"("error in (no error)"=w812, "Message Data"=w829, "Message"="Set Configuration", "Message Queue"=w845) -> ("error out"=w846:errorcluster)  [unwired: 7 out]
        n324 = Merge Errors(w846, w826) -> (w842:errorcluster)
        n325 = Cancel Notification(0:w808, 3:w842) -> (8:w871:refnum<notifier>, 11:w847:errorcluster)  [unwired: 1 out]
        n326 = Wait on Notification(notifier=w871, error in (no error)=w847) -> (notification=w869:variant, error out=w868:errorcluster)  [unwired: 4 out]
        n327 = Variant To Data(error in=w868, type=T24 {"Intensity"=[], "Wavelength"=[], "Energy"=[], "Raman Shift"=[], "Detector Temperature"=0.0} ("Measurement"), Variant=w869) -> (data=w851:T24, error out=w811:errorcluster)
        n328 = call "Measurement.vi"() -> ("Measurement"=w850:T85)
        n329 = Bundle By Name(cluster=w850, "Optical Spectrum"=w851, "Which Instrument?"=WhichInstrument."Spectrometer") -> (w852:T85)
        n330 = Cancel Notification(0:w809, 3:w811) -> (8:w807:refnum<notifier>, 11:w810:errorcluster)  [unwired: 1 out]
        n331 = Unbundle By Name(w834) -> ("Plot Data"=w853:refnum<queue>)
        n332 = call "Enqueue Message (Single).vi"("error in (no error)"=w810, "Message Data"=w852, "Message"="Append Measurement", "Message Queue"=w853) -> ("error out"=w818:errorcluster)  [unwired: 7 out]
        n333 = Unbundle By Name(w832) -> ("Instrument Sequence.Status"=w861:refnum<notifier>)
        n334 = Unbundle By Name(w832) -> ("Instrument Sequence.Measurement"=w859:refnum<notifier>)
        n335 = Unbundle By Name(w834) -> ("Optical Spectrometer"=w866:refnum<queue>)
        n336 = call "Wait for event.vi"("error in (no error)"=w810, "String"="Optical Spectrum Updated", "Notifier in"=w807) -> ("error out"=w820:errorcluster, "Notifier out"=w814:refnum<notifier>)  [unwired: 7 in]
        n337 = Cancel Notification(0:w814, 3:w820) -> (8:w813:refnum<notifier>, 11:w815:errorcluster)  [unwired: 1 out]
        n338 = call "Enqueue Message (Single).vi"("error in (no error)"=w847, "Message"="Acquire Spectrum", "Message Queue"=w866) -> ("error out"=w857:errorcluster)  [unwired: 1 in, 7 out]
        n339 = Send Notification(notification="Optical Spectrum Measured" ("Message"), notifier=w861, error in (no error)=w810) -> (error out=w855:errorcluster)  [unwired: 1 out]
        n340 = Send Notification(notification=w851, notifier=w859, error in (no error)=w810) -> (error out=w856:errorcluster)  [unwired: 1 out]
        n341 = Unbundle By Name(w834) -> ("Save Data"=w864:refnum<queue>)
        n342 = Unbundle By Name(w832) -> ("Switches & Mirrors.Status"=w841:refnum<notifier>)
        n343 = Build Array("Append Optical Spectrum" ("Message"), "Append Instrument Sequence Step" ("Message")) -> (w849:string[])
        n344 = Unbundle By Name(w834) -> ("Switches & Mirrors"=w838:refnum<queue>)
        n345 = call "Wait for event.vi"("error in (no error)"=w815, "String"="Instrument Sequence Step Appended", "Notifier in"=w813) -> ("error out"=w817:errorcluster)  [unwired: 7 in, 1 out]
        n346 = call "Enqueue Message (Array).vi"("error in (no error)"=w815, "Message Array"=w849, "Message Queue"=w864) -> ("error out"=w858:errorcluster)  [unwired: 7 in, 1 out]
        n347 = Merge Errors(w857, w855, w856, w858, w817, w818) -> (w836:errorcluster)
        n348 = Cancel Notification(0:w841, 3:w836) -> (8:w823:refnum<notifier>, 11:w822:errorcluster)  [unwired: 1 out]
        n349 = call "Wait for event.vi"("error in (no error)"=w822, "String"="Configuration Set", "Notifier in"=w823) -> ("error out"=w821:errorcluster)  [unwired: 7 in, 1 out]
        n350 = call "Enqueue Message (Single).vi"("error in (no error)"=w822, "Message Data"=w840, "Message"="Update Laser", "Message Queue"=w838) -> ("error out"=w839:errorcluster)  [unwired: 7 out]
        n351 = Merge Errors(w839, w821) -> (w835:errorcluster)
      }
      frame "Perform Optoelectronic Measurement" {
        w910 = T66 {"Relay VISA Session"="COM1", "Switches"={"Laser"=FALSE, "Video"=FALSE}, "Delays (ms)"={"Laser"=500, "Video"=1500}}  # Video Off
        w919 = T66 {"Relay VISA Session"="COM1", "Switches"={"Laser"=FALSE, "Video"=FALSE}, "Delays (ms)"={"Laser"=500, "Video"=1500}}  # Laser Off
        # "Data Saved in \nWorkspace by \nTools already"
        n352 = Unbundle By Name(w911) -> ("Save Data.Status"=w893:refnum<notifier>, "Optoelectronic.Measurement"=w892:refnum<notifier>, "Switches & Mirrors.Status"=w921:refnum<notifier>)
        n353 = Unbundle By Name(w889) -> ("Switches & Mirrors.Configuration.Switches.Laser"=w908:bool)
        n354 = Unbundle By Name(w889) -> ("Parameter Analyzer.Configuration.Acquisition Mode"=w890:enum32{"Sweeping Mode", "Sampling Mode"})
        n355 = Cancel Notification(0:w921, 3:w897) -> (8:w907:refnum<notifier>, 11:w894:errorcluster)  [unwired: 1 out]
        n356 = Unbundle By Name(w913) -> ("Switches & Mirrors"=w923:refnum<queue>)
        n357 = Bundle By Name(cluster=w910, "Switches.Laser"=w908) -> (w909:T66)
        n358 = call "Wait for event.vi"("error in (no error)"=w894, "String"="Configuration Set", "Notifier in"=w907) -> ("error out"=w906:errorcluster)  [unwired: 7 in, 1 out]
        n359 = call "Enqueue Message (Single).vi"("error in (no error)"=w894, "Message Data"=w909, "Message"="Set Configuration", "Message Queue"=w923) -> ("error out"=w924:errorcluster)  [unwired: 7 out]
        n360 = Merge Errors(w924, w906) -> (w877:errorcluster)
        n361 = Cancel Notification(0:w893, 3:w877) -> (8:w880:refnum<notifier>)  [unwired: 2 out]
        n362 = Cancel Notification(0:w892, 3:w877) -> (8:w945:refnum<notifier>, 11:w876:errorcluster)  [unwired: 1 out]
        n363 = Build Array("Optical Spectrum Updated", "Electrical Data Updated") -> (w879:string[])
        n364 = Wait on Notification(notifier=w945, error in (no error)=w876) -> (notification=w944:variant, error out=w943:errorcluster)  [unwired: 4 out]
        n365 = call "Wait for multiple events.vi"("error in (no error)"=w876, "Messages"=w879, "Notifier in"=w880) -> ("error out"=w874:errorcluster, "Notifier out"=w873:refnum<notifier>)  [unwired: 7 in]
        n366 = Variant To Data(error in=w943, type=T25 {"Optical Spectrum"={"Intensity"=[], "Wavelength"=[], "Energy"=[], "Raman Shift"=[], "Detector Temperature"=0.0}, "Electrical Measurement"={"Sequence"=[], "V1"=[], "V2"=[], "V3"=[], "V4"=[], "I1"=[], "I2"=[], "I3"=[], "I4"=[]}} ("Measurement"), Variant=w944) -> (data=w888:T25, error out=w875:errorcluster)
        n367 = Unbundle By Name(w888) -> ("Optical Spectrum"=w887:T24, "Electrical Measurement"=w886:T23)
        n368 = Merge Errors(w874, w875) -> (w872:errorcluster)
        n369 = call "Measurement.vi"() -> ("Measurement"=w925:T85)
        n370 = Bundle By Name(cluster=w925, "Optical Spectrum"=w887, "Electrical Measurement"=w886, "Which Instrument?"=WhichInstrument."Optoelectronic", "Measurement Mode"=w890) -> (w927:T85)
        n371 = Cancel Notification(0:w873, 3:w872) -> (8:w895:refnum<notifier>, 11:w896:errorcluster)  [unwired: 1 out]
        n372 = Unbundle By Name(w911) -> ("Instrument Sequence.Status"=w936:refnum<notifier>)
        n373 = Unbundle By Name(w911) -> ("Instrument Sequence.Measurement"=w934:refnum<notifier>)
        n374 = Unbundle By Name(w913) -> ("Plot Data"=w928:refnum<queue>)
        n375 = Unbundle By Name(w913) -> ("Optoelectronic"=w941:refnum<queue>)
        n376 = call "Enqueue Message (Single).vi"("error in (no error)"=w872, "Message Data"=w927, "Message"="Append Measurement", "Message Queue"=w928) -> ("error out"=w899:errorcluster)  [unwired: 7 out]
        n377 = call "Enqueue Message (Single).vi"("error in (no error)"=w876, "Message"="Measure", "Message Queue"=w941) -> ("error out"=w932:errorcluster)  [unwired: 1 in, 7 out]
        n378 = Send Notification(notification="Optoelectronic Spectrum Measured" ("Message"), notifier=w936, error in (no error)=w872) -> (error out=w930:errorcluster)  [unwired: 1 out]
        n379 = Send Notification(notification=w888, notifier=w934, error in (no error)=w872) -> (error out=w931:errorcluster)  [unwired: 1 out]
        n380 = Unbundle By Name(w913) -> ("Save Data"=w939:refnum<queue>)
        n381 = Unbundle By Name(w911) -> ("Switches & Mirrors.Status"=w920:refnum<notifier>)
        n382 = Build Array("Append Optical Spectrum" ("Message"), "Append Electrical Data" ("Message"), "Append Instrument Sequence Step" ("Message")) -> (w882:string[])
        n383 = Unbundle By Name(w913) -> ("Switches & Mirrors"=w917:refnum<queue>)
        n384 = call "Wait for event.vi"("error in (no error)"=w896, "String"="Instrument Sequence Step Appended", "Notifier in"=w895) -> ("error out"=w898:errorcluster)  [unwired: 7 in, 1 out]
        n385 = call "Enqueue Message (Array).vi"("error in (no error)"=w896, "Message Array"=w882, "Message Queue"=w939) -> ("error out"=w933:errorcluster)  [unwired: 7 in, 1 out]
        n386 = Merge Errors(w932, w930, w931, w933, w898, w899) -> (w915:errorcluster)
        n387 = Cancel Notification(0:w920, 3:w915) -> (8:w903:refnum<notifier>, 11:w902:errorcluster)  [unwired: 1 out]
        n388 = call "Wait for event.vi"("error in (no error)"=w902, "String"="Configuration Set", "Notifier in"=w903) -> ("error out"=w901:errorcluster)  [unwired: 7 in, 1 out]
        n389 = call "Enqueue Message (Single).vi"("error in (no error)"=w902, "Message Data"=w919, "Message"="Update Laser", "Message Queue"=w917) -> ("error out"=w918:errorcluster)  [unwired: 7 out]
        n390 = Merge Errors(w918, w901) -> (w914:errorcluster)
      }
      frame "Configure Parameter Analyzer" {
        n391 = Unbundle By Name(w969) -> ("Save Data.Status"=w958:refnum<notifier>, "Parameter Analyzer.Status"=w976:refnum<notifier>)
        n392 = Cancel Notification(0:w958, 3:w957) -> (11:w955:errorcluster)  [unwired: 2 out]
        n393 = Cancel Notification(0:w976, 3:w957) -> (11:w975:errorcluster)  [unwired: 2 out]
        n394 = Merge Errors(w955, w975) -> (w956:errorcluster)
        n395 = Unbundle By Name(w974) -> ("Parameter Analyzer.Configuration"=w973:T27)
        n396 = Variant To Data(error in=w956, type=w973, Variant=w966) -> (data=w960:T27, error out=w954:errorcluster)
        n397 = Bundle By Name(cluster=w974, "Parameter Analyzer.Configuration"=w960) -> (w961:T60)
        n398 = Unbundle By Name(w960) -> ("Acquisition Mode"=w972:enum32{"Sweeping Mode", "Sampling Mode"})
        n399 = Unbundle By Name(w969) -> ("Parameter Analyzer.Status"=w949:refnum<notifier>, "Save Data.Status"=w950:refnum<notifier>)
        n400 = case shown="\"Sweeping Mode\", Default" w972 {
          tunnel: ["Configure Sweeping" ("Message") "Configure Sampling" ("Message")] -> w971
          tunnel: ["Sweeping Configured" ("Message") "Sampling Configured" ("Message")] -> w948
          frame "Sweeping Mode", Default {
          }
          frame "Sampling Mode" {
          }
        }
        n401 = Unbundle By Name(w965) -> ("Parameter Analyzer"=w970:refnum<queue>)
        n402 = Unbundle By Name(w965) -> ("Message Handler Loop"=w963:refnum<queue>)
        n403 = call "Enqueue Message (Single).vi"("error in (no error)"=w954, "Message Data"=w960, "Message"=w971, "Message Queue"=w970) -> ("error out"=w951:errorcluster)  [unwired: 7 out]
        n404 = call "Enqueue Message (Single).vi"("error in (no error)"=w954, "Message Data"=w960, "Message"="Parameter Analyzer - Set UI", "Message Queue"=w963) -> ("error out"=w962:errorcluster)  [unwired: 7 out]
        n405 = call "Wait for event.vi"("error in (no error)"=w954, "String"=w948, "Notifier in"=w949) -> ("error out"=w952:errorcluster)  [unwired: 7 in, 1 out]
        n406 = call "Wait for event.vi"("error in (no error)"=w954, "String"="Instrument Configuration Set", "Notifier in"=w950) -> ("error out"=w953:errorcluster)  [unwired: 7 in, 1 out]
        n407 = Merge Errors(w951, w952, w953) -> (w946:errorcluster)
        n408 = Merge Errors(w962, w946) -> (w967:errorcluster)
      }
      frame "Configure Switching Matrix" {
        n409 = Unbundle By Name(w987) -> ("Save Data.Status"=w995:refnum<notifier>, "Switching Matrix.Status"=w997:refnum<notifier>)
        n410 = Cancel Notification(0:w995, 3:w993) -> (11:w994:errorcluster)  [unwired: 2 out]
        n411 = Cancel Notification(0:w997, 3:w993) -> (11:w996:errorcluster)  [unwired: 2 out]
        n412 = Merge Errors(w994, w996) -> (w992:errorcluster)
        n413 = Unbundle By Name(w1011) -> ("Swithing Matrix.Configuration"=w1010:T38)
        n414 = Variant To Data(error in=w992, type=w1010, Variant=w1006) -> (data=w998:T38, error out=w984:errorcluster)
        n415 = Bundle By Name(cluster=w1011, "Swithing Matrix.Configuration"=w998) -> (w1000:T60)
        n416 = Unbundle By Name(w1003) -> ("Message Handler Loop"=w1002:refnum<queue>)
        n417 = Unbundle By Name(w1003) -> ("Switching Matrix"=w1008:refnum<queue>)
        n418 = call "Enqueue Message (Single).vi"("error in (no error)"=w984, "Message Data"=w998, "Message"="Set Connections", "Message Queue"=w1008) -> ("error out"=w986:errorcluster)  [unwired: 7 out]
        n419 = call "Enqueue Message (Single).vi"("error in (no error)"=w984, "Message Data"=w998, "Message"="Switching Matrix - Set UI", "Message Queue"=w1002) -> ("error out"=w1001:errorcluster)  [unwired: 7 out]
        n420 = Unbundle By Name(w987) -> ("Save Data.Status"=w989:refnum<notifier>, "Switching Matrix.Status"=w991:refnum<notifier>)
        n421 = call "Wait for event.vi"("error in (no error)"=w984, "String"="Instrument Configuration Set", "Notifier in"=w989) -> ("error out"=w985:errorcluster)  [unwired: 7 in, 1 out]
        n422 = call "Wait for event.vi"("error in (no error)"=w984, "String"="Connections Set", "Notifier in"=w991) -> ("error out"=w983:errorcluster)  [unwired: 7 in, 1 out]
        n423 = Merge Errors(w1001, w986, w985, w983) -> (w1005:errorcluster)
      }
      frame "Configure Optical Spectrometer" {
        n424 = Unbundle By Name(w1018) -> ("Save Data.Status"=w1026:refnum<notifier>, "Optical Spectrometer.Status"=w1028:refnum<notifier>)
        n425 = Cancel Notification(0:w1026) -> (11:w1025:errorcluster)  [unwired: 1 in, 2 out]
        n426 = Cancel Notification(0:w1028, 3:w1024) -> (11:w1027:errorcluster)  [unwired: 2 out]
        n427 = Merge Errors(w1025, w1027) -> (w1023:errorcluster)
        n428 = Unbundle By Name(w1046) -> ("Optical Spectrometer.Configuration"=w1035:T42, "Switches & Mirrors.Configuration.Switches"=w1034:T67)
        n429 = Bundle("Configuration"=w1035, "Switches"=w1034) -> (w1033:cluster{"Configuration":T42, "Switches":T67})  [unwired: 1 in]
        n430 = Variant To Data(error in=w1023, type=w1033, Variant=w1042) -> (data=w1032:cluster{"Configuration":T42, "Switches":T67}, error out=w1014:errorcluster)
        n431 = Unbundle By Name(w1032) -> ("Switches"=w1030:T67, "Configuration"=w1031:T42)
        n432 = Bundle By Name(cluster=w1046, "Switches & Mirrors.Configuration.Switches"=w1030, "Optical Spectrometer.Configuration"=w1031) -> (w1036:T60)
        n433 = Unbundle By Name(w1039) -> ("Optical Spectrometer"=w1044:refnum<queue>)
        n434 = Unbundle By Name(w1039) -> ("Message Handler Loop"=w1038:refnum<queue>)
        n435 = call "Enqueue Message (Single).vi"("error in (no error)"=w1014, "Message Data"=w1031, "Message"="Complete Configuration", "Message Queue"=w1044) -> ("error out"=w1016:errorcluster)  [unwired: 7 out]
        n436 = call "Enqueue Message (Single).vi"("error in (no error)"=w1014, "Message Data"=w1031, "Message"="LabramHR - Set UI", "Message Queue"=w1038) -> ("error out"=w1037:errorcluster)  [unwired: 7 out]
        n437 = Unbundle By Name(w1018) -> ("Save Data.Status"=w1020:refnum<notifier>, "Optical Spectrometer.Status"=w1022:refnum<notifier>)
        n438 = call "Wait for event.vi"("error in (no error)"=w1014, "String"="Instrument Configuration Set", "Notifier in"=w1020) -> ("error out"=w1017:errorcluster)  [unwired: 7 in, 1 out]
        n439 = call "Wait for event.vi"("error in (no error)"=w1014, "String"="Spectrometer Configured", "Notifier in"=w1022) -> ("error out"=w1015:errorcluster)  [unwired: 7 in, 1 out]
        n440 = Merge Errors(w1037, w1016, w1017, w1015) -> (w1041:errorcluster)
      }
      frame "Focus" {
        w1058 = T66 {"Relay VISA Session"="COM1", "Switches"={"Laser"=FALSE, "Video"=TRUE}, "Delays (ms)"={"Laser"=500, "Video"=1500}}  # Laser OFF Video ON
        n441 = Unbundle By Name(w1050) -> ("Switches & Mirrors.Status"=w1063:refnum<notifier>)
        n442 = Unbundle By Name(w1051) -> ("Switches & Mirrors"=w1065:refnum<queue>)
        n443 = Cancel Notification(0:w1063, 3:w1057) -> (8:w1062:refnum<notifier>, 11:w1061:errorcluster)  [unwired: 1 out]
        n444 = call "Wait for event.vi"("error in (no error)"=w1061, "String"="Configuration Set", "Notifier in"=w1062) -> ("error out"=w1060:errorcluster)  [unwired: 7 in, 1 out]
        n445 = call "Enqueue Message (Single).vi"("error in (no error)"=w1061, "Message Data"=w1058, "Message"="Set Configuration", "Message Queue"=w1065) -> ("error out"=w1066:errorcluster)  [unwired: 7 out]
        n446 = Merge Errors(w1066, w1060) -> (w1056:errorcluster)
        n447 = Unbundle By Name(w1054) -> ("AutoFocus.Configuration"=w1055:T54)
        n448 = Unbundle By Name(w1050) -> ("AutoFocus.Status"=w1069:refnum<notifier>)
        n449 = while {
          tunnel: w1069 -> [w1081]
          tunnel: w1051 -> [w1090]
          shift-right: [w1078] -> w1049
          shift-left: w1056 -> [w1089]
          shift-right: [w1087] -> w1052
          shift-left: w1055 -> [w1083]
          tunnel: w1055 -> [w1075]
          stop <- w1085 stop-if-true
          # "Using Low Resolution?"
          n450 = Cancel Notification(0:w1081, 3:w1089) -> (11:w1088:errorcluster)  [unwired: 2 out]
          n451 = while {
            shift-right: [w1162] -> w1079
            shift-left: w1088 -> [w1164]
            tunnel: [w1148] -> w1082
            tunnel: w1081 -> [w1153]
            tunnel: [w1153] -> w1080
            stop <- w1154 stop-if-true
            n452 = Wait on Notification(notifier=w1153, error in (no error)=w1164) -> (notification=w1160:variant, error out=w1163:errorcluster)  [unwired: 4 out]
            n453 = Variant To Data(error in=w1163, type="", Variant=w1160) -> (data=w1148:string, error out=w1162:errorcluster)
            n454 = Equal?(x="Focus Failed", y=w1148) -> (x = y?=w1156:bool)
            n455 = Equal?(x="Focus Corrected (Change Direction)", y=w1148) -> (x = y?=w1155:bool)
            n456 = Equal?(x="Focus Corrected (Same Direction)", y=w1148) -> (x = y?=w1152:bool)
            n457 = Equal?(x="Focus Corrected", y=w1148) -> (x = y?=w1151:bool)
            n458 = Equal?(x="Focus at Edge", y=w1148) -> (x = y?=w1149:bool)
            n459 = Compound Arithmetic op=OR(w1156, w1155, w1152, w1151, w1149) -> (w1154:bool)
          }
          n460 = Unbundle By Name(w1090) -> ("AutoFocus"=w1091:refnum<queue>)
          n461 = call "Enqueue Message (Single).vi"("error in (no error)"=w1088, "Message Data"=w1083, "Message"="Focus", "Message Queue"=w1091) -> ("error out"=w1076:errorcluster)  [unwired: 7 out]
          n462 = Unbundle By Name(w1083) -> ("Z Scan Parameters.Initial Direction"=w1086:enum16{"Up", "Down"}, "Z Scan Parameters.Z Range"=w1084:ext, "Z Scan Parameters.Resolution"=w1074:dbl)
          n463 = Unbundle By Name(w1075) -> ("Z Scan Parameters.Resolution"=w1073:dbl)
          n464 = Merge Errors(w1076, w1079) -> (w1077:errorcluster)
          n465 = Greater?(x=w1074, y=w1073) -> (0:w1072:bool)
          n466 = case shown="\"Focus Corrected (Same Direction)\", Default" w1082 {
            tunnel: w1083 -> [_ _ w1138 _]
            tunnel: [w1099 w1120 w1137 w1146] -> w1087
            tunnel: w1086 -> [w1100 _ _ _]
            tunnel: [w1098 w1119 w1134 FALSE ("x > y?")] -> w1085
            tunnel: w1075 -> [w1097 w1120 w1133 w1146]
            tunnel: w1084 -> [_ _ w1132 _]
            tunnel: w1080 -> [w1096 w1118 _ _]
            tunnel: w1077 -> [w1095 w1117 w1131 w1145]
            tunnel: [w1094 w1116 w1131 w1145] -> w1078
            tunnel: w1074 -> [_ _ w1129 _]
            tunnel: w1072 -> [w1093 w1115 _ _]
            frame "Focus Corrected (Change Direction)" {
              n467 = case "Low Resolution?" shown="False" w1093 {
                tunnel: w1100 -> [w1109 _]
                tunnel: [w1108 w1114] -> w1099
                tunnel: [TRUE FALSE] -> w1098
                tunnel: w1097 -> [w1105 w1114]
                tunnel: w1096 -> [w1103 _]
                tunnel: w1095 -> [w1102 w1113]
                tunnel: [w1101 w1113] -> w1094
                frame False {
                  # "Focus Good to Go"
                  # "Switch Z-Scan Direction"
                  n468 = case shown="\"Up\"" w1109 {
                    tunnel: [enum16{"Up", "Down"}."Up" ("Initial Direction") enum16{"Up", "Down"}."Down" ("Initial Direction")] -> w1107
                    frame "Down" {
                    }
                    frame "Up" {
                    }
                  }
                  n469 = Bundle By Name(cluster=w1105, "Z Scan Parameters.Initial Direction"=w1107) -> (w1108:T54)
                  n470 = call "Wait for event.vi"("error in (no error)"=w1102, "String"="Alignment Completed", "Notifier in"=w1103) -> ("error out"=w1101:errorcluster)  [unwired: 7 in, 1 out]
                }
                frame True {
                  # "Repeat Once Again"
                }
              }
            }
            frame "Focus Corrected (Same Direction)", Default {
              n471 = case "Low Resolution?" shown="False" w1115 {
                tunnel: [TRUE FALSE] -> w1119
                tunnel: w1118 -> [w1123 _]
                tunnel: w1117 -> [w1122 w1127]
                tunnel: [w1121 w1127] -> w1116
                frame False {
                  # "Focus Good to Go"
                  n472 = call "Wait for event.vi"("error in (no error)"=w1122, "String"="Alignment Completed", "Notifier in"=w1123) -> ("error out"=w1121:errorcluster)  [unwired: 7 in, 1 out]
                }
                frame True {
                  # "Repeat Focus Once Again"
                }
              }
            }
            frame "Focus Failed" {
              w1130 = ext 2.0 ("x")
              n473 = Greater?(x=w1132, y=ext 100.0) -> (0:w1134:bool)
              n474 = Multiply(x=w1130, y=w1129) -> (x*y=w1128:ext)
              n475 = Multiply(x=w1130, y=w1132) -> (x*y=w1136:ext)
              n476 = case shown="False" w1134 {
                tunnel: w1138 -> [w1142 _]
                tunnel: [w1141 w1143] -> w1137
                tunnel: w1136 -> [w1140 _]
                tunnel: w1133 -> [_ w1143]
                tunnel: w1128 -> [w1139 _]
                frame False {
                  n477 = Bundle By Name(cluster=w1142, "Z Scan Parameters.Z Range"=w1140, "Z Scan Parameters.Resolution"=w1139) -> (w1141:T54)
                }
                frame True {
                }
              }
            }
            frame "Focus at Edge" {
              # "Just Repeat the Focus Procedure \nonce more with the initial Focus\nparameters"
            }
          }
        }
        n478 = Bundle By Name(cluster=w1054, "AutoFocus.Configuration"=w1052) -> (w1053:T60)
      }
      frame "Stop Sequence" {
        n479 = Unbundle By Name(w1168) -> ("Instrument Sequence"=w1167:refnum<queue>)
        n480 = Flush Queue(queue=w1167, error in (no error)=w1170) -> (error out=w1165:errorcluster)  [unwired: 2 out]
      }
      frame "Pause Sequence" {
        n481 = Unbundle By Name(w1178) -> ("Pause-Resume"=w1176:refnum<vi>)
        n482 = call "Pause.vi"("error in (no error)"=w1179, "Pause-Resume"=w1176) -> ("error out"=w1177:errorcluster)  [unwired: 9 out]
      }
      frame "Declare Completion" {
        w1192 = "Instrument Sequence Completed" ("message")
        n483 = Unbundle By Name(w1187) -> ("Instrument Sequence.Status"=w1186:refnum<notifier>)
        n484 = case shown="\"Stress Measurement VI\"" w1188 {
          tunnel: [w1200 w1201] -> w1191
          tunnel: w1192 -> [w1199 _]
          tunnel: w1189 -> [w1198 w1201]
          frame "User", Default {
            n485 = call "Dialog.vi"("error in (no error)"=w1198, "message"=w1199) -> ("error out"=w1200:errorcluster)  [unwired: 1 in, 8 out]
          }
          frame "Stress Measurement VI" {
          }
        }
        n486 = Send Notification(notification=w1192, notifier=w1186, error in (no error)=w1191) -> (error out=w1190:errorcluster)  [unwired: 1 out]
      }
    }
  }
  "error out" <- w6
  "Instrument Steps" <- w4
